vi "Dashboard Main.vi"() -> ()   [LabVIEW 2017]
uses:
  <vilib>/Utility/miscctls.llb/LVRowAndColumnTypeDef.ctl
  <vilib>/event_ctls.llb/eventvkey.ctl
  <vilib>/Rock Robotics/Network Tables/NT Read Numeric Array.vi
  <vilib>/Rock Robotics/WPI/Dashboard/WPI_DashboardLogging Global.vi
  <vilib>/Utility/config.llb/Read Key (Double).vi
  <vilib>/Utility/config.llb/Read Key (I32).vi
  <vilib>/Utility/config.llb/Write Key (Double).vi
  <vilib>/Utility/config.llb/Write Key (I32).vi
  <vilib>/Rock Robotics/Network Tables/NT Write Boolean.vi
  <vilib>/Utility/config.llb/NI_LVConfig.lvlib
panel:
  in  "Camera Settings Right":T1={"Frame Rate"=30, "Compression"=30, "Size"=1, "DB Camera Config"=FALSE} {"Frame Rate" scale=1.0..30.0; "Compression" scale=100.0..-1.0; "Size" items=["640x480", "320x240", "160x120"]}
  in  "Camera Name Right":string(combo)="No Camera Selection"
  out "Camera Info":cluster{"Mbps LED":bool, "Mbps":dbl, "fps":dbl} {"fps" format="%#.1g"; "Mbps" format="%#.1g"}
  in  "Camera Settings":T1={"Frame Rate"=30, "Compression"=30, "Size"=1, "DB Camera Config"=FALSE} {"Frame Rate" scale=1.0..30.0; "Compression" scale=100.0..-1.0; "Size" items=["640x480", "320x240", "160x120"]}
  in  "TCP":refnum<k5>
  in  "Rec Mode":enum32{"Stop", "Record", "Playback"}(radio)
  out "Robot IP":string
  out "Image Message":string="Timeout in Camera Communications"
  in  "Dashboard Tab":T2(tab)
  in  "DriveMode":T3(ring)
  in  "Autonomous":enum16{"CrossTheLine", "DoNothing"}(ring)
  in  "Encoders":T4(radio)
  in  "RobotPosition":T5(ring)
  in  "Gyro":bool
  in  "Boolean 2":bool
  in  "Select Auto":string(combo)="Select Autonomous ..."
  out "NT Connection":bool
  out "MotorChart R":cluster{"Numeric":dbl, "Numeric":dbl}(graph)
  out "MotorChart L":cluster{"Numeric":dbl, "Numeric":dbl}(graph)
  out "MotorSliders R":cluster{"MotorSlide1":dbl, "MotorSlide2":dbl} {"MotorSlide2" scale=-1.0..1.0 scale format="%#_2e"; "MotorSlide1" scale=-1.0..1.0 scale format="%#_2e"}
  out "MotorSliders L":cluster{"MotorSlide1":dbl, "MotorSlide2":dbl} {"MotorSlide2" scale=-1.0..1.0 scale format="%#_2e"; "MotorSlide1" scale=-1.0..1.0 scale format="%#_2e"}
  out "Gyro":dbl(knob) scale=0.0..360.0
  out "JS1 Z":dbl(slide) scale=-1.0..1.0 scale format="%#_2e"
  out "JS1 Graph":cluster{"X":dbl, "Y":dbl}[](graph)
  out "JS1 Buttons":T6
  out "JS2 Z":dbl(slide) scale=-1.0..1.0 scale format="%#_2e"
  out "JS2 Graph":cluster{"X":dbl, "Y":dbl}[](graph)
  out "JS2 Buttons":T6
  out "Mode":T7(ring)=enum."Auto Disabled"
  in  "ConfigFile":enum16{"Competition", "Sister", "DrivePractice"}(ring)
  out "Camera Image Right":T8(plugin-control)
  in  "Load":bool
  in  "Save":bool
  in  "DAutoGyro":dbl
  in  "IAutoGyro":dbl
  in  "PAutoGyro":dbl
  in  "FAutoGyro":dbl
  in  "RampRateAuto":dbl
  in  "FAutoRight":dbl
  in  "DAuto":dbl
  in  "IAuto":dbl
  in  "PAuto":dbl
  in  "FAutoLeft":dbl
  in  "DTeleGyro":dbl
  in  "ITeleGyro":dbl
  in  "PTeleGyro":dbl
  in  "RampRateTele":dbl
  in  "XYRatio":dbl
  in  "NormalPercent":dbl
  in  "TurboPercent":dbl
  in  "DriveMaxRPM":dbl
  in  "DTele":dbl
  in  "ITele":dbl
  in  "PTele":dbl
  in  "FTeleRight":dbl
  in  "FTeleLeft":dbl
  in  "FTeleGyro":dbl
  in  "Logging":bool
  in  "Test Slider":dbl(slide) scale=0.0..100.0 scale format="%#_3g"
  in  "On/Off":bool caption="Solenoid"
  in  "Test Name":u16(ring) items=["Select the test to run..."]
  in  "Test Tree":string(tree)
  in  "Motor":cluster{"Value":dbl, "Enable":bool} {"Value" scale=-1.0..1.0 scale format="%#_3g"}
  out "Progress":T9 {"Test Progress" scale=0.0..100.0}
  in  "Rev/Fwd":cluster{"Forward":bool, "Reverse":bool}
  in  "Test Ring":u16(ring) items=["Monochrome", "Color"]
  out "Cmd Status":string
  in  "Execute Command":bool
  in  "Command Params":string[][](table)
  in  "Command Selection":i32(listbox)
  in  "CheckList":i32(listbox)
  out "Tree":string(tree)
  out "Camera Image":T8(plugin-control)
  out "Background":bool
  in  "Camera Name":string(combo)="No Camera Selection"
  # "HW"
  # "HW"
  # "Joysticks"
  # "Front"
  # "Drive Motors"
  # "Right"
  # "Left"
  # "Back"
  # "This tab is a great place for autonomous settings and robot-specific values.\nPlace controls and indicators inside this tab and match name to\nDashboard Variables on robot. You can also delete this comment."
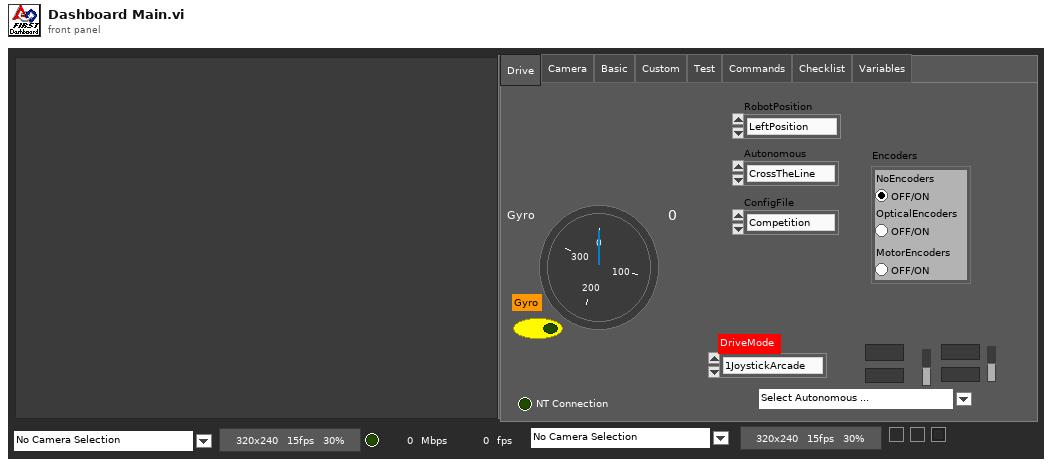
[diagram p1: front panel]
types:
  T1 = cluster{"Frame Rate":i32, "Compression":i32, "Size":u16, "DB Camera Config":bool}
  T2 = enum32{"Drive", "Camera", "Basic", "Custom", "Test", "Commands", "Checklist", "Variables"}
  T3 = enum16{"1JoystickArcade", "2JoystickArcade", "Tank"}
  T4 = enum32{"NoEncoders", "OpticalEncoders", "MotorEncoders"}
  T5 = enum16{"LeftPosition", "MiddlePosition", "RightPosition"}
  T6 = cluster{bool, bool, bool, bool, bool, bool, bool, bool, bool, bool, bool, bool}
  T7 = enum8{"Tele-Op Disabled", "Tele-Op Enabled", "Auto Disabled", "Auto Enabled", "Test Disabled", "Test Enabled", "Disconnected", "No Code", "E-Stop"}
  T8 = typedef "IMAQ Image.ctl" = refnum<image>
  T9 = cluster{"Test Progress":u8, "Test Progress Text":string}
  T10 = cluster{"Save Path":path, "Interval (s)":dbl, "Keep":i32}
  T11 = typedef "Image Type" = u32
  T12 = cluster{"IDs":cluster{"RPC field ID":u16, "Unique ID":u16}, "String":string}
  T13 = cluster{"Error Strings":string, "Disable Counts":cluster{u16, u16}, "Rail Faults":cluster{u16, u16, u16}, "Robot IP":string, "DB Mode":u8, "Event Info":cluster{"Name":string, "Type":u8, "Number":u16, "Replay":u8}}
  T14 = cluster{"Storage":cluster{"Disk Free":u64, "RAM Block":u32, "RAM free":u32}, "CPU Utilization":cluster{"CPU % ISR":sgl, "CPU % Time Crit":sgl, "CPU % Timed Str":sgl, "CPU % High":sgl, "CPU % Above":sgl, "CPU % Normal":sgl, "CPU % Low":sgl}, "CAN":cluster{"% Bus Utilization":sgl, "Bus Off Cnt":u32, "TX_FIFO Full Cnt":u32, "Receive Error Cnt":u8, "Transmit Error Cnt":u8}, "HID":cluster{"HID Outputs":u32, "Rumble Low":u16, "Rumble High":u16}[]}
  T15 = cluster{"Status bits":cluster{"Test Mode":bool, "Autonomous":bool, "Enabled":bool, "Code Start":bool, "Brownout":bool, "Reserved 2":bool, "Reserved 3":bool, "E-Stop":bool}, "Code Trace":cluster{"Disabled":bool, "TeleOp":bool, "Auto":bool, "Test":bool}, "Controller Type":enum16{"unknown", "cRIO", "roboRio"}, "Code?":enum16{"unknown", "noCode", "code"}, "Battery V":dbl}
  T16 = cluster{"Control Bits":cluster{"TestMode":bool, "Autonomous":bool, "Enabled":bool, "FMS Present":bool, bool, bool, bool, "E-Stop":bool}, "Team Station ":u8, "Countdown":sgl, "Joystick Values":cluster{"Axes":dbl[], "Buttons":bool[], "POVs":i16[]}[]}
  T17 = cluster{"Axes":dbl[], "Buttons":bool[], "POVs":i16[]}[]
  T18 = cluster{"Axes":dbl[], "Buttons":bool[], "POVs":i16[]}
  T19 = cluster{"Buttons[0]":bool, "Buttons[1]":bool, "Buttons[2]":bool, "Buttons[3]":bool, "Buttons[4]":bool, "Buttons[5]":bool, "Buttons[6]":bool, "Buttons[7]":bool, "Buttons[8]":bool, "Buttons[9]":bool, "Buttons[10]":bool, "Buttons[11]":bool}
  T20 = cluster{"Camera Name":string, string, "Saved DB Images Info":cluster{"Save Path":path, "Interval (s)":dbl, "Keep":i32}}
  T21 = cluster{"Camera Name Right":string, string, "Saved DB Images Info":cluster{"Save Path":path, "Interval (s)":dbl, "Keep":i32}}
  T22 = cluster{"Operation":enum16{"Update", "Clear"}, "Color Box":u32}[]
  T23 = typedef "eventvkey.ctl" = enum16{"ASCII", "Enter", "Return", "Shift", "Ctrl", "Alt", "Cmd", "Opt", "Caps", "NumLock", "Clear", "Break", "Up", "Down", "Left", "Right", "Insert", "Delete", "Home", "End", "PageUp", "PageDown", "Escape", "Help", "Pause", "ScrollLock", "F1", "F2", "F3", "F4", "F5", "F6", "F7", "F8", "F9", "F10", "F11", "F12", "F13", "F14", "F15", "F16", "F17", "F18", "F19", "F20", "F21", "F22", "F23", "F24", "Play", "VolumeUp", "VolumeDown", "Mute", "Two Byte Char"}
  T24 = cluster{"Image Size":bool, "Image Type":bool, "Pixel Value":bool, "ROI Information":bool, "Zoom Factor":bool}
  T25 = cluster{"Operation":enum16{"Update", "Clear"}, "Color Box":u32}
  T26 = typedef "LVRowAndColumnTypeDef.ctl" = cluster{"Row":i32, "Column":i32}
  T27 = cluster{"Shift":bool, "Ctrl":bool, "Alt":bool, "Cmd":bool, "Opt":bool}
  T28 = typedef "NI_LVConfig.lvlib/Config Data RefNum.ctl" = refnum<k1>
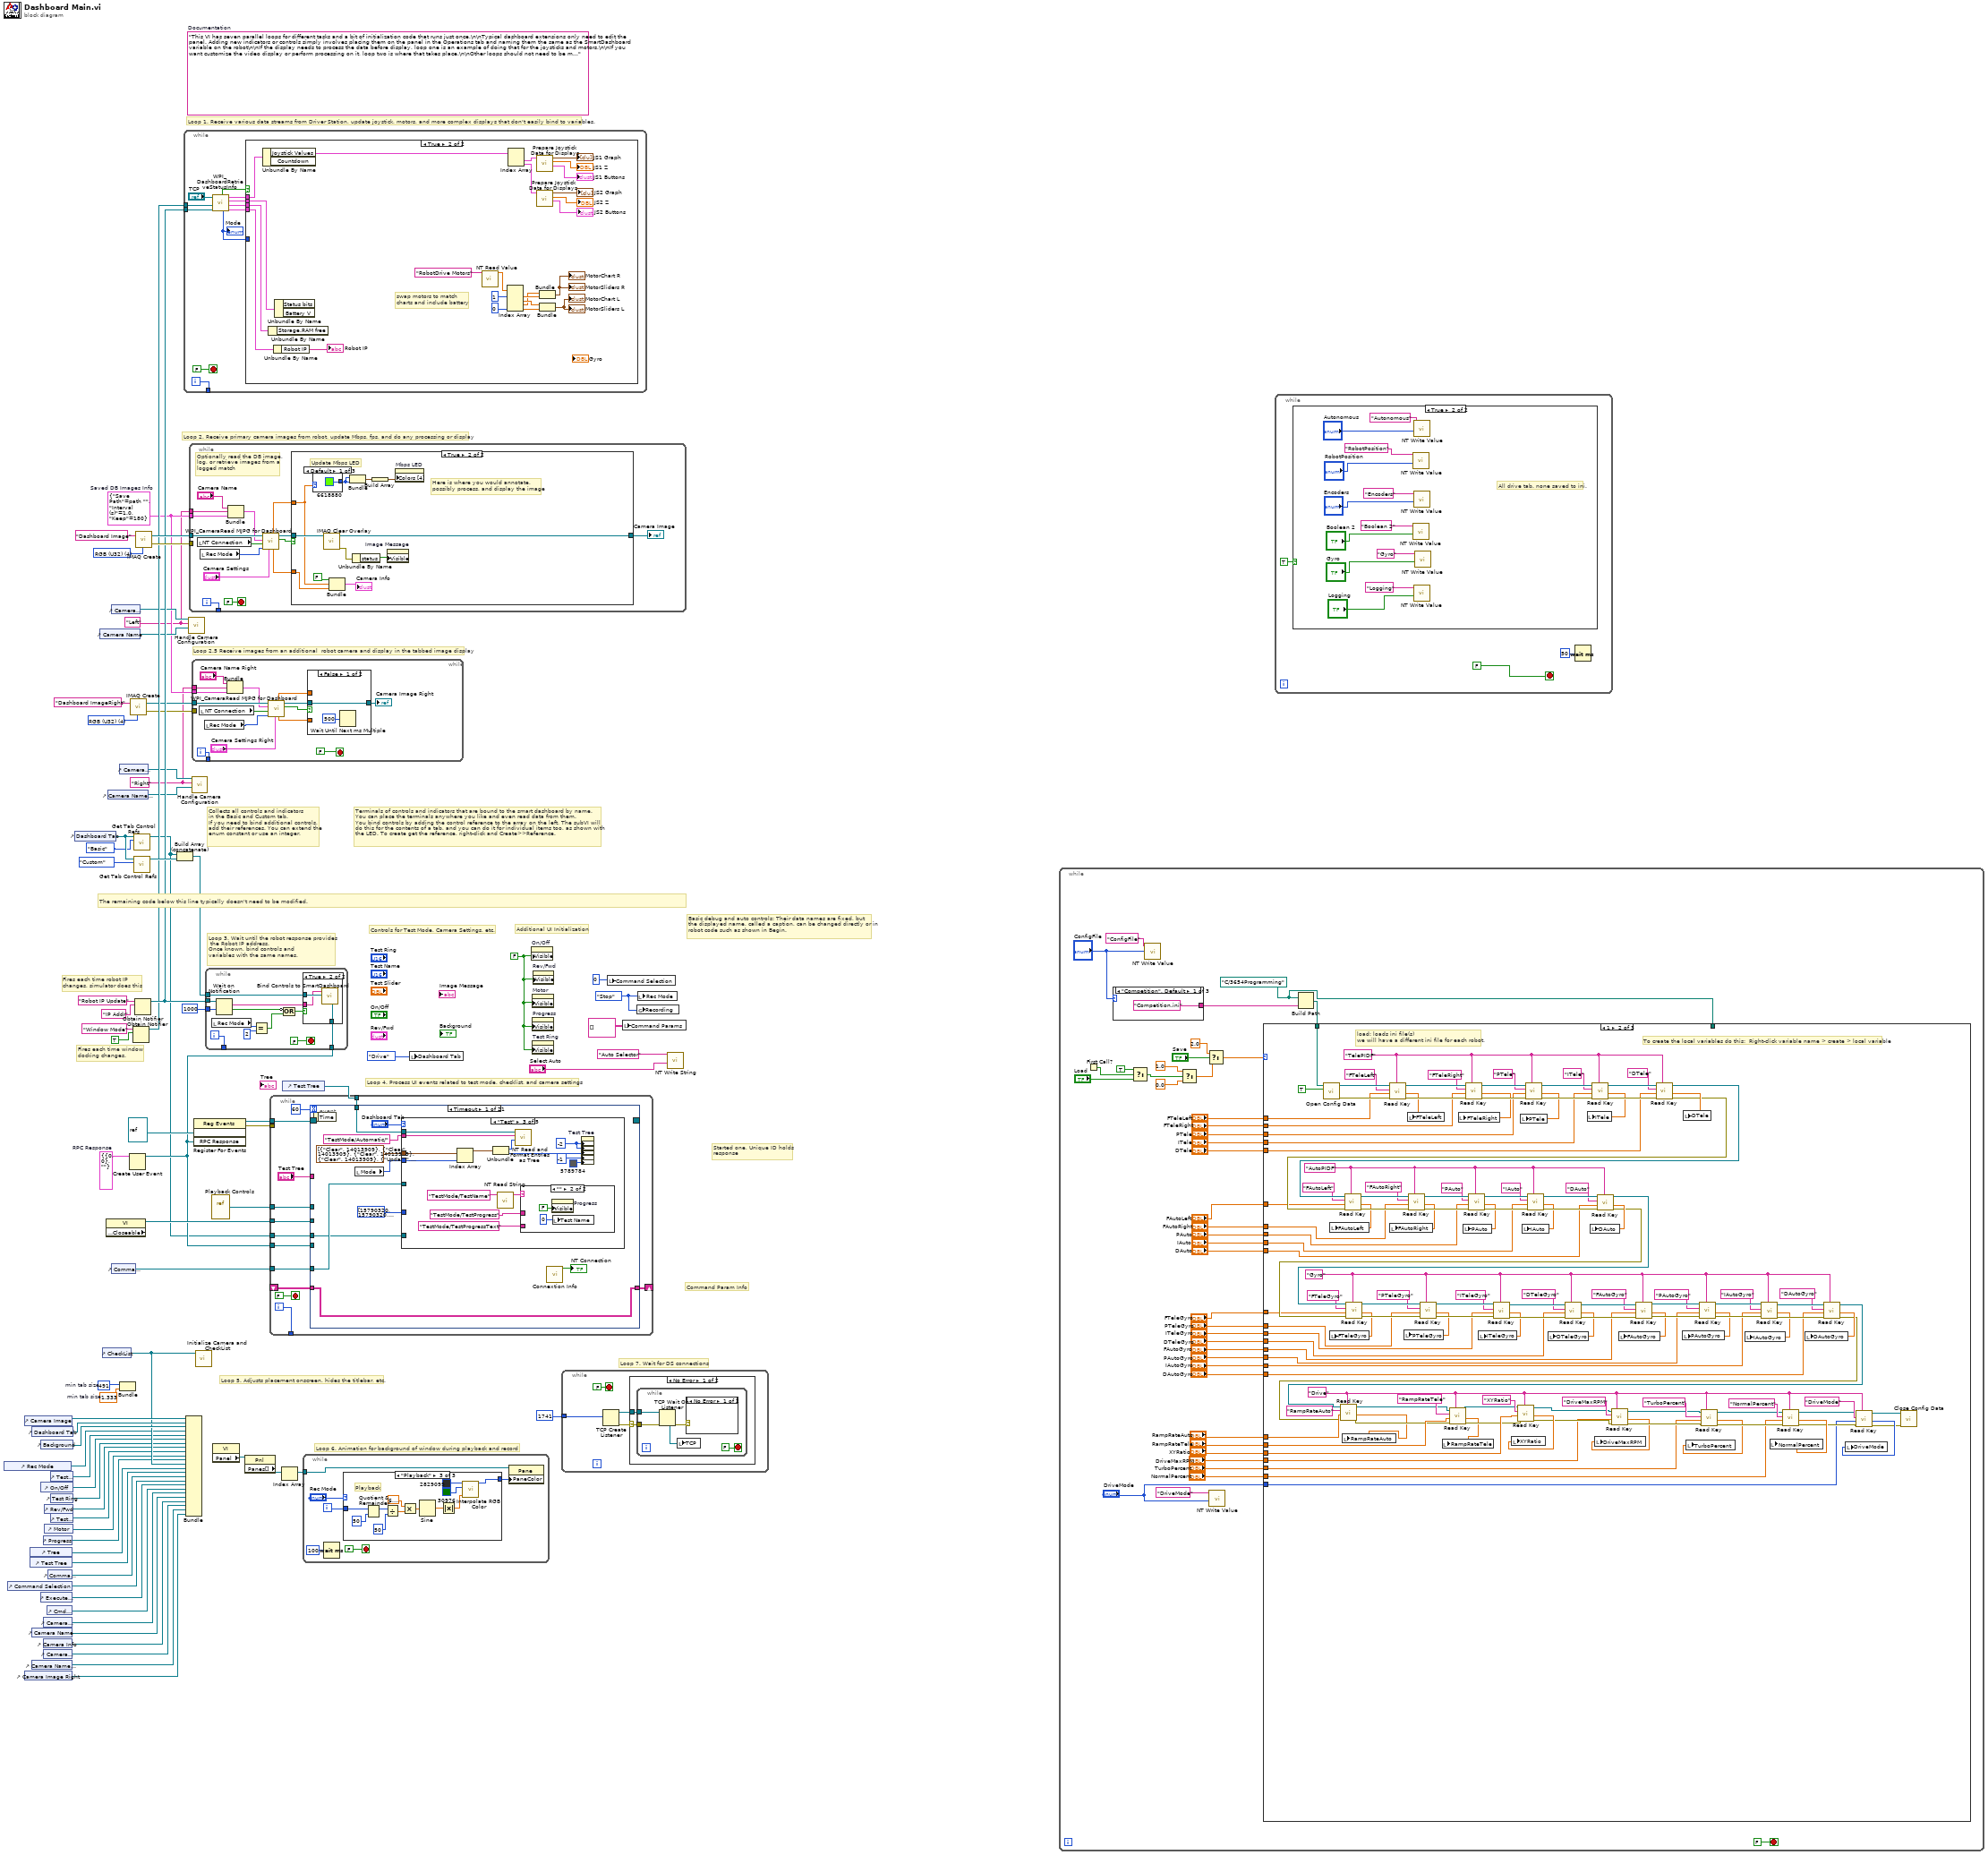
[diagram p0: block diagram]
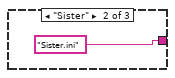
[diagram p3: hidden frame]
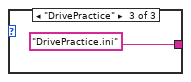
[diagram p4: hidden frame]
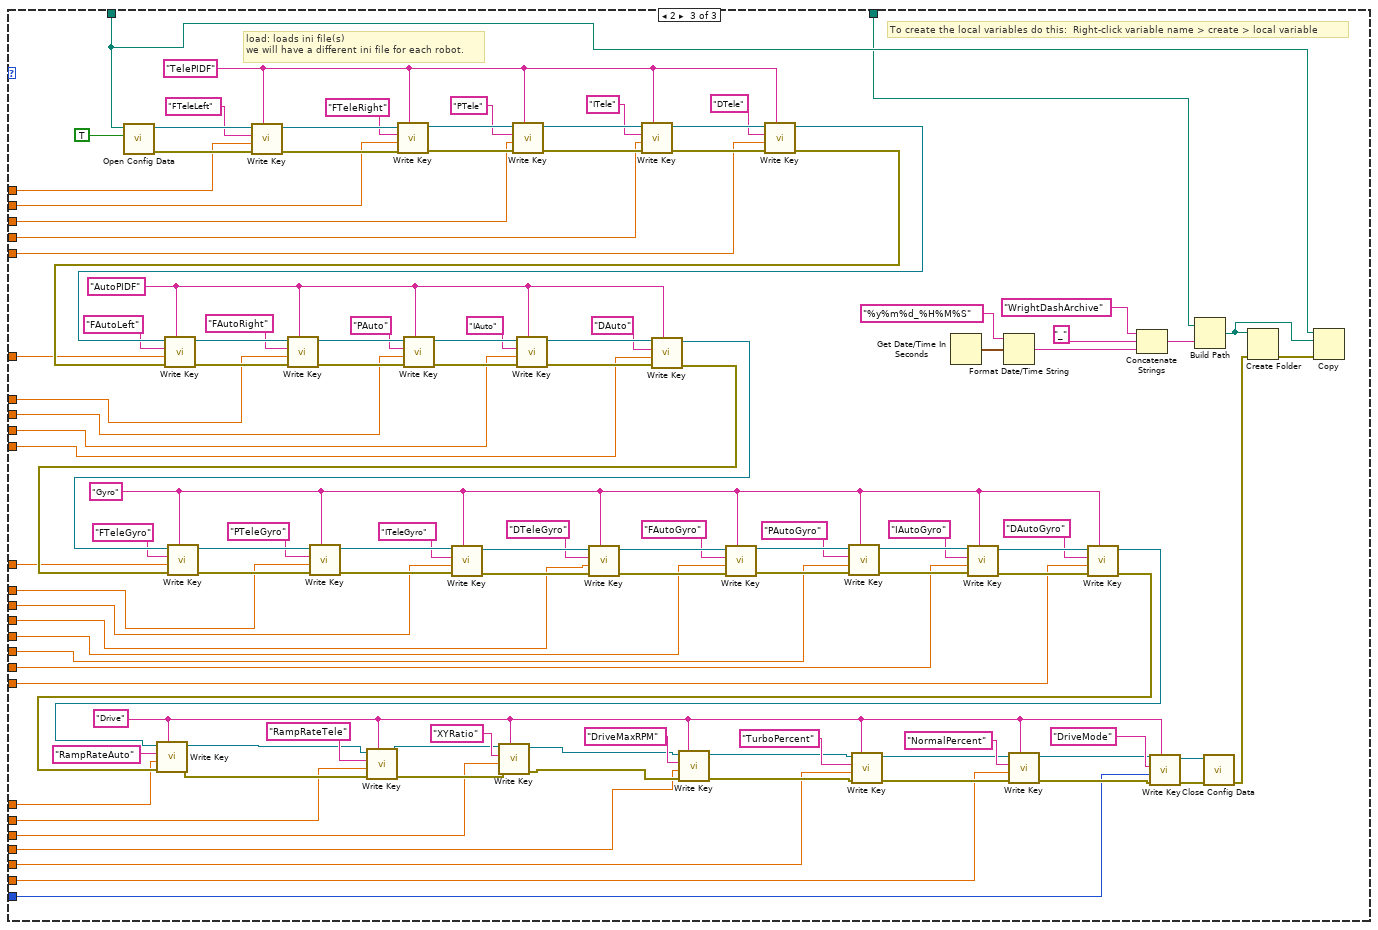
[diagram p6: hidden frame]
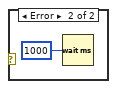
[diagram p8: hidden frame]
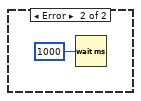
[diagram p9: hidden frame]
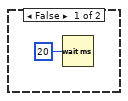
[diagram p10: hidden frame]
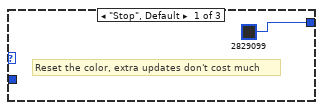
[diagram p11: hidden frame]
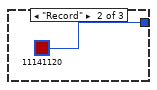
[diagram p12: hidden frame]
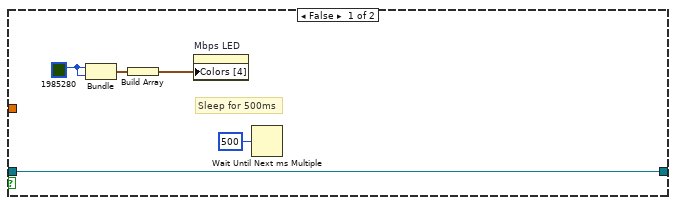
[diagram p14: hidden frame]
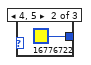
[diagram p15: hidden frame]
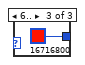
[diagram p16: hidden frame]
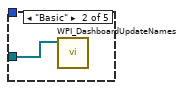
[diagram p18: hidden frame]
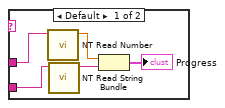
[diagram p19: hidden frame]
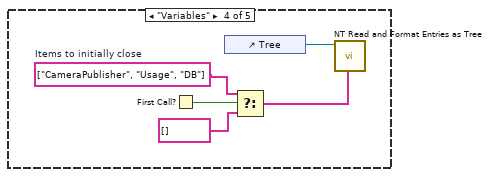
[diagram p20: hidden frame]
diagram:
  w3 = T10 {"Save Path"=path "", "Interval (s)"=1.0, "Keep"=180}  # Saved DB Images Info
  w2 = "Right"
  w1 = "Left"
  w13 = T11 4 items=["Grayscale (U8)", "Grayscale (I16)", "Grayscale (SGL)", "Complex (CSG)", "RGB (U32)", "HSL (U32)", "RGB (U64)"] ("Image Type")
  w29 = T12 {"IDs"={"RPC field ID"=0, "Unique ID"=0}, "String"=""}  # RPC Response
  w50 = 491  # min tab size
  w49 = 1.333  # min tab size
  w57 = enum32{"Stop", "Record", "Playback"}."Stop" ("Rec Mode")
  w36 = FALSE ("Visible")
  (unwired) "This VI has seven parallel loops for different tasks and a bit of initialization code that runs just once.\n\nTypical dashboard extensions only need to edit the panel. Adding new indicators or controls simply involves placing them on the panel in the Operations tab and naming them the same as the SmartDashboard variable on the robot\n\nIf the display needs to process the data before display, loop one is an example of doing that for the joysticks and motors.\n\nIf you want customize the video display or perform processing on it, loop two is where that takes place.\n\nOther loops should not need to be modified. They are pretty standard, and document the task they perform."  # Documentation
  w74 = T11 4 items=["Grayscale (U8)", "Grayscale (I16)", "Grayscale (SGL)", "Complex (CSG)", "RGB (U32)", "HSL (U32)", "RGB (U64)"] ("Image Type")
  # "Loop 2.5 Receive images from an additional  robot camera and display in the tabbed image display"
  # "Command Param Info"
  # "Started one, Unique ID holds\nresponse"
  # "Loop 7. Wait for DS connections"
  # "Basic debug and auto controls: Their data names are fixed, but\nthe displayed name, called a caption, can be changed directly or in\nrobot code such as shown in Begin."
  # "Controls for Test Mode, Camera Settings, etc."
  # "Additional UI Initialization"
  # "Loop 6. Animation for background of window during playback and record"
  # "Fires each time robot IP\nchanges, simulator does this"
  # "Fires each time window\ndocking changes."
  # "Collects all controls and indicators\nin the Basic and Custom tab.\nIf you need to bind additional controls,\nadd their references. You can extend the\nenum constant or use an integer."
  # "The remaining code below this line typically doesn't need to be modified."
  # "Loop 4. Process UI events related to test mode, checklist, and camera settings"
  # "Terminals of controls and indicators that are bound to the smart dashboard by name.\nYou can place the terminals anywhere you like and even read data from them.\nYou bind controls by adding the control reference to the array on the left. The subVI will\ndo this for the contents of a tab, and you can do it for individual items too, as shown with\nthe LED. To create get the reference, right-click and Create>>Reference."
  # "Loop 3. Wait until the robot response provides\n the Robot IP address.\nOnce known, bind controls and\nvariables with the same names."
  # "Loop 5. Adjusts placement onscreen, hides the titlebar, etc."
  # "Loop 1. Receive various data streams from Driver Station, update joystick, motors, and more complex displays that don't easily bind to variables."
  # "Loop 2. Receive primary camera images from robot, update Mbps, fps, and do any processing or display"
  n1 = control-ref of="Rec Mode"() -> (w42:refnum<vi>)
  n2 = control-ref of="Command Selection"() -> (w28:refnum<vi>)
  n3 = control-ref of="Camera Image Right"() -> (w6:refnum<vi>)
  n4 = control-ref of="Camera Image"() -> (w52:refnum<vi>)
  n5 = control-ref of="Tree"() -> (w46:refnum<vi>)
  n6 = control-ref of="Test Tree"() -> (w45:refnum<vi>)
  n7 = control-ref of="Dashboard Tab"() -> (w51:refnum<vi>)
  n8 = control-ref of="Camera Name"() -> (w19:refnum<vi>)
  n9 = control-ref of="Camera Name Right"() -> (w7:refnum<vi>)
  n10 = control-ref of="Execute Command"() -> (w30:refnum<vi>)
  n11 = control-ref of="Background"() -> (w48:refnum<vi>)
  n12 = control-ref of="On/Off"() -> (w40:refnum<vi>)
  n13 = control-ref of="Progress"() -> (w37:refnum<vi>)
  n14 = control-ref of="Camera Settings"() -> (w20:refnum<vi>)
  n15 = control-ref of="Camera Info"() -> (w18:refnum<vi>)
  n16 = control-ref of="Camera Settings Right"() -> (w8:refnum<vi>)
  n17 = control-ref of="Rev/Fwd"() -> (w38:refnum<vi>)
  n18 = control-ref of="Motor"() -> (w43:refnum<vi>)
  n19 = control-ref of="Cmd Status"() -> (w24:refnum<vi>)
  n20 = control-ref of="Command Params"() -> (w31:refnum<vi>)
  n21 = control-ref of="Test Slider"() -> (w41:refnum<vi>)
  n22 = control-ref of="Test Ring"() -> (w39:refnum<vi>)
  n23 = control-ref of="Test Name"() -> (w44:refnum<vi>)
  n24 = control-ref of="Dashboard Tab"() -> (w55:refnum<vi>)
  n25 = control-ref of="Camera Name"() -> (w21:refnum<vi>)
  n26 = control-ref of="CheckList"() -> (w47:refnum<vi>)
  n27 = property class="VI" props=["Front Panel.Closeable"]() -> (reference out=w56:refnum<vi>)  [unwired: 2 in, 2 out]
  n28 = control-ref of="Camera Name Right"() -> (w9:refnum<vi>)
  n29 = control-ref of="Camera Settings"() -> (w22:refnum<vi>)
  n30 = control-ref of="Command Params"() -> (w23:refnum<vi>)
  n31 = control-ref of="Camera Settings Right"() -> (w10:refnum<vi>)
  n32 = Bundle("min tab size"=w50, "min tab size"=w49) -> ()  [unwired: 1 in, 1 out]
  n33 = Create User Event(user event datatype=w29) -> (user event=w25:refnum<user-event>)  [unwired: 1 in, 1 out]
  n34 = call "IMAQ Create"("Image Name"="Dashboard ImageRight", "Image Type"=w13) -> ("New Image"=w12:T8, "error out"=w11:errorcluster)  [unwired: 2 in, 1 out]
  n35 = Obtain Notifier(name (unnamed)="Window Mode", notification data type=TRUE) -> (notifier out=w34:refnum<notifier>)  [unwired: 2 in, 2 out]
  n36 = call <vilib>:"Get Tab Control Refs.vi"("Page Index"=T2."Basic" ("Dashboard Tab"), "TabControl in"=w55) -> ("ControlsOnPage"=w17:refnum<vi>[])  [unwired: 9 in]
  n37 = call <vilib>:"Get Tab Control Refs.vi"("Page Index"=T2."Custom" ("Dashboard Tab"), "TabControl in"=w55) -> ("ControlsOnPage"=w54:refnum<vi>[])  [unwired: 9 in]
  n38 = Obtain Notifier(name (unnamed)="Robot IP Update", notification data type="IP Addr" ("name (unnamed)")) -> (notifier out=w35:refnum<notifier>)  [unwired: 2 in, 2 out]
  n39 = call "IMAQ Create"("Image Name"="Dashboard Image", "Image Type"=w74) -> ("New Image"=w72:T8, "error out"=w71:errorcluster)  [unwired: 2 in, 1 out]
  n40 = Build Array (concatenate)(w17, w54) -> (w53:refnum<vi>[])
  n41 = while {
    tunnel: [w84] -> _
    tunnel: w35 -> [w78]
    tunnel: w34 -> [w75]
    i -> [w84]
    stop <- FALSE stop-if-true
    n42 = call <vilib>:"WPI_DashboardRetrieveStatusInfo.vi"("Binding Refnum"=w78, "Window Mode Notifier"=w75, "TCP Cnx"="TCP") -> ("Power and Errors"=w79:T13, "Robot Metrics"=w82:T14, "Status Info"=w83:T15, "Control Info"=w80:T16, "Robot Mode"=w77:T7, "Process?"=w81:bool)  [unwired: 3 in]
    "Mode" <- w77
    n43 = case shown="True" w81 {
      tunnel: w83 -> [_ w110]
      tunnel: w82 -> [_ w109]
      tunnel: w80 -> [_ w108]
      tunnel: w79 -> [_ w107]
      tunnel: w77 -> [_ _]
      frame False {
        n44 = Wait (ms)(milliseconds to wait=u32 20) -> ()  [unwired: 1 out]
      }
      frame True {
        # "swap motors to match\ncharts and include battery"
        n45 = Unbundle By Name(w108) -> ("Joystick Values"=w98:T17)  [unwired: 1 out]
        n46 = Unbundle By Name(w109) -> ()  [unwired: 1 out]
        n47 = Unbundle By Name(w107) -> ("Robot IP"=→"Robot IP":string)
        n48 = Unbundle By Name(w110) -> ()  [unwired: 2 out]
        n49 = call-poly <vilib>:"NT Read Value.vi"("Name"="RobotDrive Motors") -> ("Numeric Array"=w88:dbl[])  [unwired: 9 in, 1 out]
        n50 = Index Array(array=w88, index #1=1, index #4=0) -> (element #1=w102:dbl, element #2=w103:dbl, element #3=w101:dbl, element #4=w106:dbl)  [unwired: 2 in]
        n51 = Index Array(array=w98) -> (element #1=w97:T18, element #2=w93:T18)  [unwired: 2 in]
        n52 = call "Prepare Joystick Data for Displays.vi"("Joystick Values"=w93) -> ("Buttons"=→"JS2 Buttons":T19, "Z Axis"=→"JS2 Z":dbl, "Cartesian Data"=→"JS2 Graph":cluster{"X axis":dbl, "X axis":dbl}[])  [unwired: 8 in]
        n53 = call "Prepare Joystick Data for Displays.vi"("Joystick Values"=w97) -> ("Buttons"=→"JS1 Buttons":T19, "Z Axis"=→"JS1 Z":dbl, "Cartesian Data"=→"JS1 Graph":cluster{"X axis":dbl, "X axis":dbl}[])  [unwired: 8 in]
        n54 = Bundle("Numeric"=w101, "Numeric"=w102) -> (→"MotorChart R" →"MotorSliders R":cluster{"Numeric":dbl, "Numeric":dbl})  [unwired: 1 in]
        n55 = Bundle("Numeric"=w103, "Numeric"=w106) -> (→"MotorChart L" →"MotorSliders L":cluster{"Numeric":dbl, "Numeric":dbl})  [unwired: 1 in]
      }
    }
  }
  n56 = Bundle("Camera Image"=w52, "Dashboard Tab"=w51, "Background"=w48, "Rec Mode"=w42, "Test Slider"=w41, "On/Off"=w40, "Test Ring"=w39, "Rev/Fwd"=w38, "Test Name"=w44, "Motor"=w43, "Progress"=w37, "CheckList"=w47, "Tree"=w46, "Test Tree"=w45, "Command Params"=w31, "Command Selection"=w28, "Execute Command"=w30, "Cmd Status"=w24, "Camera Settings"=w20, "Camera Name"=w19, "Camera Info"=w18, "Camera Settings Right"=w8, "Camera Name Right"=w7, "Camera Image Right"=w6) -> ()  [unwired: 1 in, 1 out]
  n57 = call "Handle Camera Configuration.vi"("CameraNameRef"=w21, "Display Name"=w1, "ClusterRef"=w22) -> ()  [unwired: 9 in]
  n58 = while {
    tunnel: w72 -> [w123]
    tunnel: w71 -> [_]
    tunnel: [w124] -> _
    tunnel: w3 -> [w114]
    tunnel: w1 -> [w111]
    i -> [w124]
    stop <- FALSE stop-if-true
    # "Optionally read the DB image,\nlog, or retrieve images from a\nlogged match"
    n59 = local read "NT Connection"() -> (w115:bool)
    n60 = local read "Rec Mode"() -> (w119:enum32{"Stop", "Record", "Playback"})
    n61 = Bundle("Camera Name"="Camera Name", w111, "Saved DB Images Info"=w114) -> (w113:T20)  [unwired: 1 in]
    n62 = call <vilib>:"WPI_CameraRead MJPG for Dashboard.vi"("Camera Settings"="Camera Settings", "Rec Mode"=w119, "NT Connection"=w115, "Capture Info"=w113, "Refnum in"=w123) -> ("Active"=w121:bool, "Refnum out"=w122:T8, "FPS"=w120:dbl, "Bandwidth (Mbps)"=w118:dbl)  [unwired: 3 in]
    n63 = case shown="True" w121 {
      tunnel: w122 -> [w126 w137]
      tunnel: w118 -> [_ w134]
      tunnel: w120 -> [_ w135]
      tunnel: [w126 w131] -> w116
      frame False {
        w128 = u32 1985280 ("Color Box")
        # "Sleep for 500ms"
        n64 = Bundle("Color Box"=w128, "Color Box"=w128) -> (w129:cluster{"Color Box":u32, "Color Box":u32})  [unwired: 1 out]
        n65 = Build Array(w129) -> (w127:cluster{"Color Box":u32, "Color Box":u32}[])
        n66 = property on="Mbps LED" class="Bool (strict)"("Colors [4]"=w127) -> ()  [unwired: 2 in, 2 out]
        n67 = Wait Until Next ms Multiple(millisecond multiple=u32 500) -> ()  [unwired: 1 out]
      }
      frame True {
        # "Here is where you would annotate,\npossibly process, and display the image"
        # "Update Mbps LED"
        n68 = case shown="Default" w134 {
          tunnel: [u32 6618880 ("Color Box") u32 16776722 ("Color Box") u32 16716800 ("Color Box")] -> w138
          frame Default {
          }
          frame 4, 5 {
          }
          frame 6.. {
          }
        }
        n69 = call "IMAQ Clear Overlay"("Image"=w137) -> ("error out"=w140:errorcluster, "Image Out"=w131:T8)  [unwired: 2 in, 7 out]
        n70 = Bundle(FALSE, "Bandwidth (Mbps)"=w134, "FPS"=w135) -> (→"Camera Info":cluster{bool, "Bandwidth (Mbps)":dbl, "FPS":dbl})  [unwired: 1 in]
        n71 = Bundle("Color Box"=w138, "Color Box"=w138) -> (w139:cluster{"Color Box":u32, "Color Box":u32})  [unwired: 1 out]
        n72 = Unbundle By Name(w140) -> ("status"=w141:bool)
        n73 = Build Array(w139) -> (w136:cluster{"Color Box":u32, "Color Box":u32}[])
        n74 = property on="Image Message" class="Str"("Visible"=w141) -> ()  [unwired: 2 in, 2 out]
        n75 = property on="Mbps LED" class="Bool (strict)"("Colors [4]"=w136) -> ()  [unwired: 2 in, 2 out]
      }
    }
    "Camera Image" <- w116
  }
  n76 = call "Handle Camera Configuration.vi"("CameraNameRef"=w9, "Display Name"=w2, "ClusterRef"=w10) -> ()  [unwired: 9 in]
  n77 = while {
    tunnel: w12 -> [w159]
    tunnel: w11 -> [_]
    tunnel: [w154] -> _
    tunnel: w3 -> [w148]
    tunnel: w2 -> [w145]
    i -> [w154]
    stop <- FALSE stop-if-true
    n78 = local read "NT Connection"() -> (w149:bool)
    n79 = local read "Rec Mode"() -> (w158:enum32{"Stop", "Record", "Playback"})
    n80 = Bundle("Camera Name Right"="Camera Name Right", w145, "Saved DB Images Info"=w148) -> (w147:T21)  [unwired: 1 in]
    n81 = call <vilib>:"WPI_CameraRead MJPG for Dashboard.vi"("Camera Settings"="Camera Settings Right", "Rec Mode"=w158, "NT Connection"=w149, "Capture Info"=w147, "Refnum in"=w159) -> ("Active"=w153:bool, "Refnum out"=w156:T8, "FPS"=w151:dbl, "Bandwidth (Mbps)"=w152:dbl)  [unwired: 3 in]
    n82 = case shown="False" w153 {
      tunnel: w156 -> [w160 w162]
      tunnel: w152 -> [_ _]
      tunnel: w151 -> [_ _]
      tunnel: [w160 w162] -> w150
      frame False {
        n83 = Wait Until Next ms Multiple(millisecond multiple=u32 500) -> ()  [unwired: 1 out]
      }
      frame True {
      }
    }
    "Camera Image Right" <- w150
  }
  n84 = register-events(refnum<vi> refnum, w25) -> (reference out=w61:refnum<event-registration>, error out=w60:errorcluster)  [unwired: 2 in]
  n85 = call "Initialize Camera and CheckList.vi"("ListBox in"=w47) -> ()  [unwired: 11 in]
  n86 = while {
    tunnel: w53 -> [w174]
    tunnel: w35 -> [w172]
    tunnel: [w170] -> _
    tunnel: u32 1000 ("milliseconds to wait") -> [w169]
    tunnel: w25 -> [w163]
    i -> [w170]
    stop <- FALSE stop-if-true
    n87 = local read "Rec Mode"() -> (w165:enum32{"Stop", "Record", "Playback"})
    n88 = Wait on Notification(notifier=w172, timeout in ms (-1)=w169) -> (notification=w171:string, timed out?=w167:bool)  [unwired: 2 in, 2 out]
    n89 = Equal?(x=w165, y=u16 2 ("Rec Mode")) -> (x = y?=w166:bool)
    n90 = Compound Arithmetic op=OR(invert w167, w166) -> (w168:bool)
    n91 = case shown="True" w168 {
      tunnel: w174 -> [_ w177]
      tunnel: w171 -> [_ w176]
      tunnel: w163 -> [_ w175]
      frame False {
      }
      frame True {
        n92 = call <vilib>:"Bind Controls to SmartDashboard.vi"("RPC ref"=w175, "Bound Control Refs"=w177, "Server IP Address"=w176) -> ()  [unwired: 9 in]
      }
    }
  }
  n93 = vi-ref "Playback Controls.vi"() -> (w62:refnum<vi>)
  n94 = property class="VI"() -> ("Panel"=w64:refnum<vi>)  [unwired: 2 in, 2 out]
  n95 = property class="Pnl"(reference=w64) -> ("Panes[]"=w65:refnum<vi>[])  [unwired: 1 in, 2 out]
  n96 = Index Array(array=w65) -> (element=w63:refnum<vi>)  [unwired: 1 in]
  n97 = control-ref of="Test Tree"() -> (w66:refnum<vi>)
  n98 = while {
    tunnel: [w187] -> _
    tunnel: w66 -> [w186]
    tunnel: w62 -> [w185]
    tunnel: w61 -> [w184]
    tunnel: w60 -> [_]
    tunnel: w56 -> [w183]
    tunnel: w25 -> [w182]
    tunnel: w23 -> [w181]
    shift-right: [w180] -> _
    shift-left: _ -> [w179]
    tunnel: w17 -> [w178]
    i -> [w187]
    stop <- FALSE stop-if-true
    n99 = event shown="[0] Timeout" {
      selector: w184 -> [_ _ _ _ _ _ _ _ _ _ _ _ _ _ _ _ _ _ _ _ _]
      dyn-events: [_ _ _ _ _ _ _ _ _ _ _ _ _ _ _ _ w447 _ _ _ _] -> _
      timeout: u32 60 ("milliseconds to wait") -> [_ _ _ _ _ _ _ _ _ _ _ _ _ _ _ _ _ _ _ _ _]
      tunnel: w186 -> [w199 _ _ _ _ _ _ _ _ _ _ _ _ _ _ _ _ _ _ _ _]
      tunnel: "Test Tree" -> [_ _ _ _ _ _ _ _ _ _ _ w414 w422 w424 w428 w436 _ _ _ _ _]
      tunnel: w185 -> [_ _ _ _ _ _ _ _ _ _ _ _ _ _ _ _ w449 _ w467 _ _]
      tunnel: w183 -> [_ _ _ _ _ _ _ _ _ _ _ _ _ _ _ _ w445 _ _ _ _]
      tunnel: w182 -> [_ _ _ _ _ _ _ _ _ _ _ _ _ _ _ _ w443 _ _ _ _]
      tunnel: w181 -> [w194 _ _ _ _ _ w365 _ _ _ _ _ _ _ _ _ _ _ _ _ _]
      tunnel: [w193 w242 w344 w349 w358 w362 w363 w372 w382 w389 w401 w413 w420 w423 w427 w435 w442 w462 w464 w468 w481] -> w180
      tunnel: w179 -> [w193 w242 w344 w349 w358 w362 w363 _ _ w389 w401 w413 w420 w423 w427 w435 w442 w462 w464 w468 w481]
      tunnel: w178 -> [w191 _ _ _ _ _ _ _ _ _ _ _ _ _ _ _ _ _ _ _ _]
      event Timeout {
        n100 = event-data() -> ()  [unwired: 1 in, 1 out]
        n101 = local read "Mode"() -> (w196:T7)
        n102 = case shown="\"Test\"" "Dashboard Tab" {
          tunnel: w199 -> [_ _ w215 _ _]
          tunnel: "TestMode/Automatic/" ("Name Pattern") -> [_ _ w214 _ _]
          tunnel: T22 [{"Operation"=enum."Clear", "Color Box"=14013909}, {"Operation"=enum."Clear", "Color Box"=14013909}, {"Operation"=enum."Clear", "Color Box"=14013909}, {"Operation"=enum."Clear", "Color Box"=14013909}, {"Operation"=enum."Update", "Color Box"=14013909}, {"Operation"=enum."Update", "Color Box"=16777215}, {"Operation"=enum."Clear", "Color Box"=14013909}, {"Operation"=enum."Clear", "Color Box"=14013909}, {"Operation"=enum."Clear", "Color Box"=14013909}] -> [_ _ w207 _ w235]
          tunnel: w196 -> [_ _ w206 _ w234]
          tunnel: u32[] [15790320, 15790320, 15790320, 15790320, 16777215, 16777215, 15790320, 15790320, 15790320] -> [_ _ _ _ w240]
          tunnel: w194 -> [_ _ _ _ w228]
          tunnel: w191 -> [_ w201 _ _ _]
          frame "Custom", Default {
          }
          frame "Basic" {
            n103 = call <vilib>:"WPI_DashboardUpdateNames.vi"("Controls on Tab"=w201) -> ()  [unwired: 11 in]
          }
          frame "Test" {
            w213 = -2 ("Active Item:Row Number")
            n104 = Index Array(array=w207, index=w206) -> (element=w208:T25)
            n105 = Unbundle(w208) -> ("Operation"=w209:enum16{"Update", "Clear"}, "Color Box"=w210:u32)
            n106 = call <vilib>:"NT Read String.vi"("Name"="TestMode/TestName") -> ("String"=w204:string)  [unwired: 9 in, 1 out]
            n107 = call <vilib>:"NT Read and Format Entries as Tree.vi"("Operation"=w209, "Name Pattern"=w214, "Tree Refnum"=w215) -> ()  [unwired: 7 in, 2 out]
            n108 = case shown="\"\"" w204 {
              tunnel: "TestMode/TestProgress" ("Name") -> [w217 _]
              tunnel: "TestMode/TestProgressText" ("Name") -> [w216 _]
              frame Default {
                n109 = call <vilib>:"NT Read Number.vi"("Name"=w217) -> ("Numeric"=w218:dbl)  [unwired: 9 in, 1 out]
                n110 = call <vilib>:"NT Read String.vi"("Name"=w216) -> ("String"=w219:string)  [unwired: 9 in, 1 out]
                n111 = Bundle("Numeric"=w218, "String"=w219) -> (→"Progress":cluster{"Numeric":dbl, "String":string})  [unwired: 1 in]
              }
              frame "" {
                n112 = property on="Progress" class="Clust (strict)"("Visible"=FALSE) -> ()  [unwired: 2 in, 2 out]
                n113 = local write "Test Name"(u16 0) -> ()
              }
            }
            n114 = property on="Test Tree" class="Tree (strict)"("Active Item Row Number"=w213, "ActiveColNum"=w213, "CellBG"=w210, "Active Item Row Number"=-1 ("Active Item:Row Number"), "CellBG"=u32 5789784 ("Color Box")) -> ()  [unwired: 2 in, 2 out]
          }
          frame "Variables" {
            w225 = string[] ["CameraPublisher", "Usage", "DB"]  # Items to initially close
            n115 = First Call?() -> (First Call?: T/F=w226:bool)
            n116 = control-ref of="Tree"() -> (w227:refnum<vi>)
            n117 = Select(t=w225, s=w226, f=string[] []) -> (s? t:f=w223:string[])
            n118 = call <vilib>:"NT Read and Format Entries as Tree.vi"("Tags to  Close"=w223, "Tree Refnum"=w227) -> ()  [unwired: 8 in, 2 out]
          }
          frame "Commands" {
            w236 = u32 5789784 ("Color Box")
            w237 = T26 {"Row"=-1, "Column"=-2} ("Active Cell:Active Cell")
            w239 = T26 {"Row"=-2, "Column"=-2} ("Active Cell:Active Cell")
            n119 = Index Array(array=w240, index=w234) -> (element=w238:u32)
            n120 = Index Array(array=w235, index=w234) -> (element=w233:T25)
            n121 = Unbundle(w233) -> ("Operation"=w232:enum16{"Update", "Clear"})  [unwired: 1 out]
            n122 = local read "Command Selection"() -> (w231:i32)
            n123 = property on="Command Selection" class="MCListbox (strict)"("ActiveCell"=w239, "CellBG"=w238, "ActiveCell"=w237, "CellBG"=w236) -> ()  [unwired: 2 in, 2 out]
            n124 = call <vilib>:"WPI_DashboardUpdate RPC Info.vi"("Operation"=w232) -> ("update"=w230:bool, "commands"=w229:string[][])  [unwired: 9 in]
            n125 = property on="Command Selection" class="MCListbox (strict)"("ItemNames"=w229) -> ()  [unwired: 2 in, 2 out]
            n126 = property on="Command Params" class="Tbl (strict)"("Active Cell"=w239, "Cell BG Color"=w238, "Active Cell"=w237, "Cell BG Color"=w236) -> ()  [unwired: 2 in, 2 out]
            n127 = call <vilib>:"WPI_DashboardUpdate Command Params.vi"("Update"=w230, "NewVal"=w231, "Commands"=w229, "Param Tbl"=w228) -> ()  [unwired: 7 in, 1 out]
          }
        }
        n128 = call <vilib>:"Connextion Info.vi"() -> ("Connected"=→"NT Connection":bool)  [unwired: 10 in, 1 out]
      }
      event "Test Tree": Value Change {
        # "Show appropriate\ncontrols"
        n129 = event-data() -> ("CtlRef"=w245:refnum<vi>, "NewVal"=w243:string)  [unwired: 1 in]
        n130 = call <vilib>:"WPI_UtilitiesGetTreeIOName.vi"("NewVal"=w243, "TreeControl in"=w245) -> ("I/O Name"=w246:string)  [unwired: 9 in]
        n131 = case shown="\"Camera\"" w246 {
          selector: w246 -> [_ w253 _ w275 w284 _]
          tunnel: w243 -> [_ _ w272 w274 _ w291]
          tunnel: cluster{string[]}[] [{["640x480", "320x240", "160x120"]}, {["Auto", "Fixed indoor", "Fixed outdoor 1", "Fixed outdoor 2", "Fixed fluorescent 1", "Fixed fluorescent 2", "Hold current"]}, {["Auto", "Flicker-free 50 Hz", "Flicker-free 60 Hz", "Hold current"]}, {["None", "Prioritize frame rate", "Prioritize image quality"]}, {["Monochrome", "Color"]}] -> [_ _ _ _ _ w290]
          frame Default {
            w248 = FALSE ("Visible")
            w247 = FALSE ("Visible")
            n132 = property on="Motor" class="Clust (strict)"("Visible"=w247) -> ()  [unwired: 2 in, 2 out]
            n133 = property on="Test Ring" class="Ring (strict)"("Visible"=w247) -> ()  [unwired: 2 in, 2 out]
            n134 = property on="Rev/Fwd" class="Clust (strict)"("Visible"=w248) -> ()  [unwired: 2 in, 2 out]
            n135 = property on="On/Off" class="Bool (strict)"("Visible"=w248) -> ()  [unwired: 2 in, 2 out]
            n136 = property on="Test Slider" class="Slide (strict)"("Visible"=w248) -> ()  [unwired: 2 in, 2 out]
          }
          frame "Analog Out", "Motor", "PWM" {
            w254 = FALSE ("Visible")
            n137 = case shown="\"Analog Out\"" w253 {
              tunnel: [1.0 ("Value") -1.0 ("Value") 0.0 ("Value")] -> w252
              tunnel: [255.0 ("Value") 1.0 ("Value") 5.0 ("Value")] -> w251
              tunnel: [128.0 ("Value") 0.0 ("Value") 0.0 ("Value")] -> w250
              tunnel: [64.0 ("Value") 0.5 ("Value") 1.0 ("Value")] -> w249
              frame "PWM" {
              }
              frame "Motor", Default {
              }
              frame "Analog Out" {
              }
            }
            n138 = property on="Motor" class="Clust (strict)"("Visible"=TRUE) -> ()  [unwired: 2 in, 2 out]
            n139 = property on="Value" class="Slide (strict)"("Value"=w250, "Scale.Minimum"=w252, "Scale.Maximum"=w251, "Scale.Increment"=w249) -> ()  [unwired: 2 in, 2 out]
            n140 = property on="On/Off" class="Bool (strict)"("Visible"=w254) -> ()  [unwired: 2 in, 2 out]
            n141 = property on="Test Slider" class="Slide (strict)"("Visible"=w254) -> ()  [unwired: 2 in, 2 out]
            n142 = property on="Test Ring" class="Ring (strict)"("Visible"=w254) -> ()  [unwired: 2 in, 2 out]
            n143 = property on="Rev/Fwd" class="Clust (strict)"("Visible"=w254) -> ()  [unwired: 2 in, 2 out]
          }
          frame "Servo" {
            w270 = FALSE ("Visible")
            n144 = call <vilib>:"NT Read Number.vi"("Name"=w272) -> ("Numeric"=w271:dbl)  [unwired: 9 in, 1 out]
            n145 = property on="Test Slider" class="Slide (strict)"("Visible"=TRUE, "Scale.Maximum"=170.0 ("Scale.Range:Maximum")) -> ()  [unwired: 2 in, 2 out]
            n146 = local write "Test Slider"(w271) -> ()
            n147 = property on="Motor" class="Clust (strict)"("Visible"=w270) -> ()  [unwired: 2 in, 2 out]
            n148 = property on="Rev/Fwd" class="Clust (strict)"("Visible"=w270) -> ()  [unwired: 2 in, 2 out]
            n149 = property on="On/Off" class="Bool (strict)"("Visible"=w270) -> ()  [unwired: 2 in, 2 out]
            n150 = property on="Test Ring" class="Ring (strict)"("Visible"=w270) -> ()  [unwired: 2 in, 2 out]
          }
          frame "Relay", "Solenoid" {
            w273 = FALSE ("Visible")
            n151 = property on="Motor" class="Clust (strict)"("Visible"=w273) -> ()  [unwired: 2 in, 2 out]
            n152 = property on="Test Slider" class="Slide (strict)"("Visible"=w273) -> ()  [unwired: 2 in, 2 out]
            n153 = Search and Replace String(input string=w274, search string="/Value  **", replace string="/Direction") -> (result string=w280:string)  [unwired: 5 in, 3 out]
            n154 = property on="Test Ring" class="Ring (strict)"("Visible"=w273) -> ()  [unwired: 2 in, 2 out]
            n155 = call <vilib>:"NT Read String.vi"("Name"=w280) -> ("String"=w278:string)  [unwired: 9 in, 1 out]
            n156 = Equal?(x="Both directions", y=w278) -> (x = y?=w276:bool)
            n157 = Not(x=w276) -> (.not. x?=w277:bool)
            n158 = property on="Rev/Fwd" class="Clust (strict)"("Visible"=w276) -> ()  [unwired: 2 in, 2 out]
            n159 = property on="On/Off" class="Bool (strict)"("Visible"=w277, "Caption.Text"=w275) -> ()  [unwired: 2 in, 2 out]
          }
          frame "Compressor", "Digital Out" {
            w283 = FALSE ("Visible")
            # "Get direction and finish"
            n160 = property on="Motor" class="Clust (strict)"("Visible"=w283) -> ()  [unwired: 2 in, 2 out]
            n161 = property on="Test Slider" class="Slide (strict)"("Visible"=w283) -> ()  [unwired: 2 in, 2 out]
            n162 = property on="Test Ring" class="Ring (strict)"("Visible"=w283) -> ()  [unwired: 2 in, 2 out]
            n163 = property on="On/Off" class="Bool (strict)"("Visible"=TRUE, "Caption.Text"=w284) -> ()  [unwired: 2 in, 2 out]
            n164 = property on="Rev/Fwd" class="Clust (strict)"("Visible"=FALSE) -> ()  [unwired: 2 in, 2 out]
          }
          frame "Camera" {
            n165 = call <vilib>:"Get Last Path Segment.vi"("String in"=w291) -> ("String out"=w292:string)  [unwired: 10 in]
            n166 = property on="On/Off" class="Bool (strict)"("Visible"=FALSE) -> ()  [unwired: 2 in, 2 out]
            n167 = property on="Motor" class="Clust (strict)"("Visible"=FALSE) -> ()  [unwired: 2 in, 2 out]
            n168 = property on="Rev/Fwd" class="Clust (strict)"("Visible"=FALSE) -> ()  [unwired: 2 in, 2 out]
            n169 = case shown="\"White Balance  **\"" w292 {
              tunnel: w291 -> [w298 w307 w316 w325 w334 _ w340]
              tunnel: w290 -> [w296 w304 w313 w322 w331 _ _]
              frame "Size  **" {
                n170 = Index Array(array=w296) -> (element=w295:cluster{string[]})  [unwired: 1 in]
                n171 = call <vilib>:"NT Read String.vi"("Name"=w298) -> ("String"=w297:string)  [unwired: 9 in, 1 out]
                n172 = Unbundle(w295) -> (w293:string[])
                n173 = Match First String(2:w293, 3:w297) -> (0:w294:i32)  [unwired: 1 out]
                n174 = property on="Test Ring" class="Ring (strict)"("Value"=w294, "Strings []"=w293) -> ()  [unwired: 2 in, 2 out]
                n175 = property on="Test Ring" class="Ring (strict)"("Visible"=TRUE) -> ()  [unwired: 2 in, 2 out]
                n176 = property on="Test Slider" class="Slide (strict)"("Visible"=FALSE) -> ()  [unwired: 2 in, 2 out]
              }
              frame "White Balance  **" {
                n177 = Index Array(array=w304, index=1) -> (element=w305:cluster{string[]})
                n178 = call <vilib>:"NT Read String.vi"("Name"=w307) -> ("String"=w306:string)  [unwired: 9 in, 1 out]
                n179 = Unbundle(w305) -> (w302:string[])
                n180 = Match First String(2:w302, 3:w306) -> (0:w301:i32)  [unwired: 1 out]
                n181 = property on="Test Ring" class="Ring (strict)"("Value"=w301, "Strings []"=w302) -> ()  [unwired: 2 in, 2 out]
                n182 = property on="Test Ring" class="Ring (strict)"("Visible"=TRUE) -> ()  [unwired: 2 in, 2 out]
                n183 = property on="Test Slider" class="Slide (strict)"("Visible"=FALSE) -> ()  [unwired: 2 in, 2 out]
              }
              frame "Exposure  **" {
                n184 = Index Array(array=w313, index=2) -> (element=w314:cluster{string[]})
                n185 = call <vilib>:"NT Read String.vi"("Name"=w316) -> ("String"=w315:string)  [unwired: 9 in, 1 out]
                n186 = Unbundle(w314) -> (w310:string[])
                n187 = Match First String(2:w310, 3:w315) -> (0:w311:i32)  [unwired: 1 out]
                n188 = property on="Test Ring" class="Ring (strict)"("Value"=w311, "Strings []"=w310) -> ()  [unwired: 2 in, 2 out]
                n189 = property on="Test Ring" class="Ring (strict)"("Visible"=TRUE) -> ()  [unwired: 2 in, 2 out]
                n190 = property on="Test Slider" class="Slide (strict)"("Visible"=FALSE) -> ()  [unwired: 2 in, 2 out]
              }
              frame "Exposure Priority  **" {
                n191 = Index Array(array=w322, index=3) -> (element=w323:cluster{string[]})
                n192 = call <vilib>:"NT Read String.vi"("Name"=w325) -> ("String"=w324:string)  [unwired: 9 in, 1 out]
                n193 = Unbundle(w323) -> (w319:string[])
                n194 = Match First String(2:w319, 3:w324) -> (0:w320:i32)  [unwired: 1 out]
                n195 = property on="Test Ring" class="Ring (strict)"("Value"=w320, "Strings []"=w319) -> ()  [unwired: 2 in, 2 out]
                n196 = property on="Test Ring" class="Ring (strict)"("Visible"=TRUE) -> ()  [unwired: 2 in, 2 out]
                n197 = property on="Test Slider" class="Slide (strict)"("Visible"=FALSE) -> ()  [unwired: 2 in, 2 out]
              }
              frame "Color Enable  **" {
                n198 = Index Array(array=w331, index=4) -> (element=w332:cluster{string[]})
                n199 = call <vilib>:"NT Read String.vi"("Name"=w334) -> ("String"=w333:string)  [unwired: 9 in, 1 out]
                n200 = Unbundle(w332) -> (w328:string[])
                n201 = Match First String(2:w328, 3:w333) -> (0:w329:i32)  [unwired: 1 out]
                n202 = property on="Test Ring" class="Ring (strict)"("Value"=w329, "Strings []"=w328) -> ()  [unwired: 2 in, 2 out]
                n203 = property on="Test Ring" class="Ring (strict)"("Visible"=TRUE) -> ()  [unwired: 2 in, 2 out]
                n204 = property on="Test Slider" class="Slide (strict)"("Visible"=FALSE) -> ()  [unwired: 2 in, 2 out]
              }
              frame Default {
                n205 = property on="Test Ring" class="Ring (strict)"("Visible"=FALSE) -> ()  [unwired: 2 in, 2 out]
                n206 = property on="Test Slider" class="Slide (strict)"("Visible"=FALSE) -> ()  [unwired: 2 in, 2 out]
              }
              frame "Brightness  **", "Color Level  **", "Compression  **", "FPS  **", "Sharpness  **" {
                n207 = call <vilib>:"NT Read Number.vi"("Name"=w340) -> ("Numeric"=w339:dbl)  [unwired: 9 in, 1 out]
                n208 = local write "Test Slider"(w339) -> ()
                n209 = property on="Test Slider" class="Slide (strict)"("Visible"=TRUE, "Scale.Maximum"=100.0 ("Scale.Range:Maximum")) -> ()  [unwired: 2 in, 2 out]
                n210 = property on="Test Ring" class="Ring (strict)"("Visible"=FALSE) -> ()  [unwired: 2 in, 2 out]
              }
            }
          }
        }
        n211 = property on="Progress" class="Clust (strict)"("Visible"=FALSE) -> ()  [unwired: 2 in, 2 out]
      }
      event "Test Name": Mouse Enter {
        # "Populate the ring with the list of tests"
        n212 = event-data() -> ()  [unwired: 1 in, 1 out]
        n213 = call <vilib>:"NT Read String Array.vi"("Name"="TestMode/TestList") -> ("String Array"=w348:string[])  [unwired: 9 in, 1 out]
        n214 = Build Array (concatenate)("Select the test to run...", w348) -> (w347:string[])
        n215 = property on="Test Name" class="Ring (strict)"("Strings []"=w347) -> ()  [unwired: 2 in, 2 out]
      }
      event "Test Name": Value Change {
        w350 = FALSE ("Visible")
        # "Tell the robot the test name to run"
        n216 = event-data() -> ("NewVal"=w354:u16)  [unwired: 1 in]
        n217 = property on="Test Name" class="Ring (strict)"() -> ("Strings []"=w355:string[])  [unwired: 2 in, 2 out]
        n218 = local write "Progress"(T9 {"Test Progress"=0, "Test Progress Text"=""} ("Progress")) -> ()
        n219 = Index Array(array=w355, index=w354) -> (element=w353:string)
        n220 = call <vilib>:"NT Write String.vi"("String"=w353, "Name"="TestMode/TestName") -> ()  [unwired: 9 in, 1 out]
        n221 = property on="Progress" class="Clust (strict)"("Visible"=TRUE) -> ()  [unwired: 2 in, 2 out]
        n222 = property on="Motor" class="Clust (strict)"("Visible"=w350) -> ()  [unwired: 2 in, 2 out]
        n223 = property on="Test Slider" class="Slide (strict)"("Visible"=w350) -> ()  [unwired: 2 in, 2 out]
        n224 = property on="On/Off" class="Bool (strict)"("Visible"=w350) -> ()  [unwired: 2 in, 2 out]
        n225 = property on="Rev/Fwd" class="Clust (strict)"("Visible"=w350) -> ()  [unwired: 2 in, 2 out]
        n226 = property on="Test Ring" class="Ring (strict)"("Visible"=w350) -> ()  [unwired: 2 in, 2 out]
      }
      event "Select Auto": Mouse Enter {
        # "Populate the combo box with the list of autonomous options"
        n227 = event-data() -> ()  [unwired: 1 in, 1 out]
        n228 = call <vilib>:"NT Read String Array.vi"("Name"="Auto List") -> ("String Array"=w357:string[])  [unwired: 9 in, 1 out]
        n229 = property on="Select Auto" class="CmbBox"("Strings[]"=w357) -> ()  [unwired: 2 in, 2 out]
      }
      event "Select Auto": Value Change {
        # "User modified the Auto Selection. Write to NT variable so robot knows."
        n230 = event-data() -> ("NewVal"=w360:string)  [unwired: 1 in]
        n231 = call <vilib>:"NT Write String.vi"("String"=w360, "Name"="Auto Selector") -> ()  [unwired: 9 in, 1 out]
      }
      event "Command Selection": Value Change {
        # "Get the params and show in table"
        n232 = event-data() -> ("NewVal"=w366:i32)  [unwired: 1 in]
        n233 = property on="Command Selection" class="MCListbox (strict)"() -> ("ItemNames"=w364:string[][])  [unwired: 2 in, 2 out]
        n234 = call <vilib>:"WPI_DashboardUpdate Command Params.vi"("NewVal"=w366, "Commands"=w364, "Param Tbl"=w365) -> ()  [unwired: 8 in, 1 out]
      }
      event "Execute Command": Value Change {
        # "Started one, Unique ID holds\nresponse"
        n235 = event-data() -> ()  [unwired: 1 in, 1 out]
        n236 = property on="Command Selection" class="MCListbox (strict)"() -> ("ItemNames"=w377:string[][])  [unwired: 2 in, 2 out]
        n237 = Index Array(array=w377, index (row)="Command Selection", index (col)=0) -> (element=w375:string)
        n238 = call <vilib>:"Invoke Commands.vi"("Command Params"="Command Params", "Function Name"=w375) -> ("Params"=w371:u8, "Started"=w370:bool)  [unwired: 7 in, 1 out]
        n239 = Array Subset(array="Command Params", length (row)=w371) -> (w372:string[][])  [unwired: 3 in]
        n240 = Select(t="Executing" ("Cmd Status"), s=w370, f="" ("Cmd Status")) -> (s? t:f=→"Cmd Status":string)
      }
      event "Command Selection": Double Click {
        n241 = event-data() -> ("Row"=w385:i32)  [unwired: 1 in]
        n242 = property on="Command Selection" class="MCListbox (strict)"() -> ("ItemNames"=w388:string[][])  [unwired: 2 in, 2 out]
        n243 = local read "Command Params"() -> (w384:string[][])
        n244 = Index Array(array=w388, index (row)=w385, index (col)=0) -> (element=w386:string)
        n245 = call <vilib>:"Invoke Commands.vi"("Command Params"=w384, "Function Name"=w386) -> ("Params"=w383:u8, "Started"=w378:bool)  [unwired: 7 in, 1 out]
        n246 = Array Subset(array=w384, length (row)=w383) -> (w382:string[][])  [unwired: 3 in]
        n247 = Select(t="Executing" ("Cmd Status"), s=w378, f="" ("Cmd Status")) -> (s? t:f=w379:string)
        n248 = local write "Cmd Status"(w379) -> ()
      }
      event "CheckList": Double Click {
        # "Shift clears all"
        # "Update symbols on the listbox"
        n249 = event-data() -> ("PlatMods.Shift"=w390:bool, "Row"=w392:i32)  [unwired: 1 in]
        n250 = case shown="True" w390 {
          tunnel: w392 -> [w396 _]
          tunnel: 1 -> [w395 _]
          frame False {
            n251 = property on="CheckList" class="LstBox (strict)"() -> ("Item Symbols"=w394:i32[])  [unwired: 2 in, 2 out]
            n252 = Replace Array Subset(array=w394, new element=w395, index=w396) -> (w393:i32[])
            n253 = property on="CheckList" class="LstBox (strict)"("Item Symbols"=w393) -> ()  [unwired: 2 in, 2 out]
          }
          frame True {
            w397 = 0 ("Top Row")
            n254 = property on="CheckList" class="LstBox (strict)"() -> ("Number of Rows"=w399:u32)  [unwired: 2 in, 2 out]
            n255 = Initialize Array(0, w399) -> (w398:i32[])
            n256 = property on="CheckList" class="LstBox (strict)"("Top Row"=w397, "Value"=w397, "Item Symbols"=w398) -> ()  [unwired: 2 in, 2 out]
          }
        }
      }
      event "CheckList": Key Down {
        # "Update symbols on the listbox\nLeft and right keys check and uncheck"
        n257 = event-data() -> ("VKey"=w403:T23)  [unwired: 1 in]
        n258 = case shown="\"Left\", \"Right\"" w403 {
          selector: w403 -> [w408 _]
          tunnel: eventvkey."Left" ("VKey") -> [w406 _]
          frame "Left", "Right" {
            n259 = Equal?(x=w406, y=w408) -> (x = y?=w407:bool)
            n260 = Select(t=0, s=w407, f=1) -> (s? t:f=w409:i32)
            n261 = property on="CheckList" class="LstBox (strict)"() -> ("Item Symbols"=w412:i32[])  [unwired: 2 in, 2 out]
            n262 = Replace Array Subset(array=w412, new element=w409, index="CheckList") -> (w411:i32[])
            n263 = property on="CheckList" class="LstBox (strict)"("Item Symbols"=w411) -> ()  [unwired: 2 in, 2 out]
          }
          frame Default {
          }
        }
      }
      event "Motor.Enable": Value Change {
        # "When the test mode otor enable helper is set, update that\ntree row item's value"
        n264 = event-data() -> ("NewVal"=w418:bool)  [unwired: 1 in]
        n265 = Unbundle("Motor") -> ("Value"=w417:dbl)  [unwired: 1 out]
        n266 = Select(t=w417, s=w418, f=0.0) -> (s? t:f=w415:dbl)
        n267 = call <vilib>:"NT Write Number.vi"("Numeric"=w415, "Name"=w414) -> ()  [unwired: 9 in, 1 out]
      }
      event "Test Slider": Value Change {
        # "When the test mode slider helper is set, update that\ntree row item's value"
        n268 = event-data() -> ("NewVal"=w421:dbl)  [unwired: 1 in]
        n269 = call <vilib>:"NT Write Number.vi"("Numeric"=w421, "Name"=w422) -> ()  [unwired: 9 in, 1 out]
      }
      event "On/Off": Value Change {
        # "When the test mode on/off helper value is set, update that\ntree row item's value"
        n270 = event-data() -> ("NewVal"=w426:bool)  [unwired: 1 in]
        n271 = Boolean To (0,1)(Boolean=w426) -> (0, 1=w425:i16)
        n272 = call <vilib>:"NT Write Number.vi"("Numeric"=w425, "Name"=w424) -> ()  [unwired: 9 in, 1 out]
      }
      event "Rev/Fwd": Value Change {
        # "When the test mode helper value for relays is set, update that\ntree row item's value"
        n273 = event-data() -> ("NewVal.Forward"=w434:bool, "NewVal.Reverse"=w433:bool)  [unwired: 1 in]
        n274 = Boolean To (0,1)(Boolean=w434) -> (0, 1=w430:i16)
        n275 = Boolean To (0,1)(Boolean=w433) -> (0, 1=w432:i16)
        n276 = Negate(x=w432) -> (-x=w431:i16)
        n277 = Add(x=w430, y=w431) -> (x+y=w429:i16)
        n278 = call <vilib>:"NT Write Number.vi"("Numeric"=w429, "Name"=w428) -> ()  [unwired: 9 in, 1 out]
      }
      event "Test Ring": Value Change {
        # "When a test mode helper value is selected from the ring,\nset the tree item's variable to the string value"
        n279 = event-data() -> ("NewVal"=w438:u16)  [unwired: 1 in]
        n280 = property on="Test Ring" class="Ring (strict)"() -> ("Strings []"=w439:string[])  [unwired: 2 in, 2 out]
        n281 = Index Array(array=w439, index=w438) -> (element=w437:string)
        n282 = call <vilib>:"NT Write String.vi"("String"=w437, "Name"=w436) -> ()  [unwired: 9 in, 1 out]
      }
      event "Rec Mode": Value Change {
        # "Update globals for recording mode and path to read log from.\nClear when logging and let NetworkTables set path for vision to\nuse."
        n283 = event-data() -> ("NewVal"=w450:enum32{"Stop", "Record", "Playback"})  [unwired: 1 in]
        n284 = global write "WPI_DashboardLogging Global.vi" "Logging Filename"(path "") -> ()
        n285 = global write "WPI_DashboardLogging Global.vi" "Recording"(w450) -> ()
        n286 = case shown="\"Playback\"" w450 {
          tunnel: w449 -> [_ w452 w461]
          tunnel: [_ _ w460] -> w447
          tunnel: [_ _ w459] -> _
          tunnel: w445 -> [_ _ w457]
          tunnel: cluster{i32, i32} {-250, 170} -> [_ _ w456]
          tunnel: [_ _ T24 {"Image Size"=TRUE, "Image Type"=TRUE, "Pixel Value"=TRUE, "ROI Information"=TRUE, "Zoom Factor"=FALSE} ("Image Information Shown:All Elements")] -> w440
          tunnel: [_ _ TRUE ("Zoom Factor")] -> w441
          tunnel: w443 -> [_ _ w453]
          frame Default {
          }
          frame "Stop", "Record" {
            # "Place Window too"
            n287 = invoke class="VI" method="FP.Close"(reference=w452) -> (reference out=w451:refnum<vi>)  [unwired: 2 in, 2 out]
            n288 = invoke class="VI" method="Abort VI"(reference=w451) -> ()  [unwired: 2 in, 3 out]
          }
          frame "Playback" {
            n289 = call "Open Playback Panel.vi"("Offset"=w456, "DB VI Ref"=w457, "Playback in"=w461) -> ("Playback out"=w458:refnum<vi>)  [unwired: 8 in]
            n290 = register-events(w458, w453) -> (reference out=w460:refnum<event-registration>, error out=w459:errorcluster)  [unwired: 2 in]
          }
        }
        n291 = property on="Camera Image Right" class="ImageControl"("Image Information Shown"=w440, "Image Information Visible"=w441) -> ()  [unwired: 2 in, 2 out]
        n292 = property on="Camera Image" class="ImageControl"("Image Information Shown"=w440, "Image Information Visible"=w441) -> ()  [unwired: 2 in, 2 out]
        n293 = call <vilib>:"WPI_DashboardNT Log FieldName Cache.vi"("Operation"=enum16{"Lookup/Add", "Index", "Clear"}."Clear") -> ()  [unwired: 8 in, 3 out]
      }
      event Panel Close {
        w463 = enum32{"Stop", "Record", "Playback"}."Stop" ("Rec Mode")
        # "Playback window has been closed, abort"
        n294 = event-data() -> ()  [unwired: 1 in, 4 out]
        n295 = local write "Rec Mode"(w463) -> ()
        n296 = global write "WPI_DashboardLogging Global.vi" "Recording"(w463) -> ()
      }
      event Panel Close {
        # "Abort playback window and ourself"
        n297 = event-data() -> ()  [unwired: 1 in, 4 out]
        n298 = invoke class="VI" method="FP.Close"(reference=w467) -> (reference out=w466:refnum<vi>)  [unwired: 2 in, 2 out]
        n299 = invoke class="VI" method="Abort VI"(reference=w466) -> (error out=w465:errorcluster)  [unwired: 2 in, 2 out]
        n300 = invoke class="VI" method="Abort VI"(error in=w465) -> ()  [unwired: 2 in, 3 out]
      }
      event User Event {
        n301 = event-data() -> ("IDs"=w474:cluster{"RPC field ID":u16, "Unique ID":u16}, "String"=w473:string)  [unwired: 1 in]
        n302 = Bundle("IDs"=w474, "String"=w473) -> (w472:T12)  [unwired: 1 in]
        n303 = call <vilib>:"Retrieve RPC Response.vi"("RPC Response"=w472) -> ("Output"=w470:string[][])  [unwired: 10 in]
        n304 = Build Array (concatenate)(w468, w470) -> (w469:string[][])
        n305 = local write "Command Params"(w469) -> ()
        n306 = local write "Cmd Status"("" ("Cmd Status")) -> ()
      }
      event "Tree": Double Click {
        n307 = event-data() -> ("PlatMods"=w480:T27, "Tag"=w477:string)  [unwired: 1 in]
        n308 = Unbundle(w480) -> ("Shift"=w479:bool)  [unwired: 4 out]
        n309 = String Subset(string=w477, length (rest)=1 ("length (rest)")) -> (substring=w476:string)  [unwired: 1 in]
        n310 = Not(x=w479) -> (.not. x?=w478:bool)
        n311 = case shown="\"/\"" w476 {
          tunnel: w477 -> [_ w483]
          tunnel: w478 -> [_ w482]
          frame Default {
          }
          frame "/" {
            n312 = call <vilib>:"NT Update Persistence.vi"("Persistence"=w482, "Name"=w483) -> ()  [unwired: 9 in, 1 out]
          }
        }
      }
    }
  }
  n313 = while {
    tunnel: w63 -> [w485]
    i -> [w488]
    stop <- FALSE stop-if-true
    n314 = Wait (ms)(milliseconds to wait=u32 100) -> ()  [unwired: 1 out]
    n315 = case shown="\"Playback\"" "Rec Mode" {
      tunnel: w488 -> [_ _ w503]
      tunnel: [u32 2829099 ("Base Color") u32 11141120 ("Target Color") w492] -> w484
      frame "Stop", Default {
        # "Reset the color, extra updates don't cost much"
      }
      frame "Record" {
      }
      frame "Playback" {
        # "Playback"
        n316 = Quotient & Remainder(x=w503, y=u32 50 ("milliseconds to wait")) -> (x-y*floor(x/y)=w499:u32)  [unwired: 1 out]
        n317 = Divide(x=w499, y=u32 50 ("milliseconds to wait")) -> (x/y=w496:dbl)
        n318 = Multiply(x=6.283185307179586, y=w496) -> (x*y=w501:dbl)
        n319 = Sine(x=w501) -> (sin(x)=w500:dbl)
        n320 = Absolute Value(x=w500) -> (abs(x)=w493:dbl)
        n321 = call "Interpolate RGB Color.vi"("Proportion"=w493, "Target Color"=u32 30976, "Base Color"=u32 2829099) -> ("Result Color"=w492:u32)  [unwired: 8 in]
      }
    }
    n322 = property class="Pane"(reference=w485, "PaneColor"=w484) -> ()  [unwired: 1 in, 2 out]
  }
  n323 = local write "Dashboard Tab"(T2."Drive" ("Dashboard Tab")) -> ()
  n324 = property on="On/Off" class="Bool (strict)"("Visible"=w36) -> ()  [unwired: 2 in, 2 out]
  n325 = property on="Motor" class="Clust (strict)"("Visible"=w36) -> ()  [unwired: 2 in, 2 out]
  n326 = property on="Progress" class="Clust (strict)"("Visible"=w36) -> ()  [unwired: 2 in, 2 out]
  n327 = property on="Test Ring" class="Ring (strict)"("Visible"=w36) -> ()  [unwired: 2 in, 2 out]
  n328 = property on="Rev/Fwd" class="Clust (strict)"("Visible"=w36) -> ()  [unwired: 2 in, 2 out]
  n329 = while {
    tunnel: u16 1741 ("timeout ms (25000)") -> [w505]
    stop <- FALSE stop-if-true
    n330 = TCP Create Listener(10:w505) -> (0:w504:errorcluster, 3:w506:refnum<k5>)  [unwired: 4 in, 1 out]
    n331 = case shown="No Error" w504 {
      selector: w504 -> [w508 _]
      tunnel: w506 -> [w509 _]
      frame No Error {
        n332 = while {
          tunnel: w509 -> [w512]
          tunnel: w508 -> [w511]
          stop <- FALSE stop-if-true
          n333 = TCP Wait On Listener(8:w511, 11:w512) -> (0:w513:errorcluster, 4:w514:refnum<k5>)  [unwired: 2 in, 3 out]
          n334 = local write "TCP"(w514) -> ()
          n335 = case shown="No Error" w513 {
            frame No Error {
            }
            frame Error {
              n336 = Wait (ms)(milliseconds to wait=u32 1000) -> ()  [unwired: 1 out]
            }
          }
        }
      }
      frame Error {
        n337 = Wait (ms)(milliseconds to wait=u32 1000) -> ()  [unwired: 1 out]
      }
    }
  }
  n338 = local write "Command Selection"(u16 0 ("milliseconds to wait")) -> ()
  n339 = local write "Command Params"(string[][] [] ("Command Params")) -> ()
  n340 = global write "WPI_DashboardLogging Global.vi" "Recording"(w57) -> ()
  n341 = local write "Rec Mode"(w57) -> ()
  n342 = call <vilib>:"NT Write String.vi"("String"="Select Auto", "Name"="Auto Selector") -> ()  [unwired: 9 in, 1 out]
  n343 = while {
    stop <- FALSE stop-if-true
    w520 = path "C:/3654Programming" ("base path")
    n344 = First Call?() -> (First Call?: T/F=w551:bool)
    n345 = case shown="\"Competition\", Default" "ConfigFile" {
      tunnel: ["Competition.ini" "Sister.ini" "DrivePractice.ini"] -> w547
      frame "Competition", Default {
      }
      frame "Sister" {
      }
      frame "DrivePractice" {
      }
    }
    n346 = Select(t=TRUE, s=w551, f="Load") -> (s? t:f=w558:bool)
    n347 = call-poly <vilib>:"NT Write Value.vi"("Numeric"="ConfigFile", "Name"="ConfigFile") -> ()  [unwired: 9 in, 1 out]
    n348 = Select(t=1.0, s=w558, f=0.0) -> (s? t:f=w557:dbl)
    n349 = Select(t=2.0, s="Save", f=w557) -> (s? t:f=w549:dbl)
    n350 = call-poly <vilib>:"NT Write Value.vi"("Numeric"="DriveMode", "Name"="DriveMode") -> ()  [unwired: 9 in, 1 out]
    n351 = Build Path(base path=w520, name or relative path=w547) -> (appended path=w546:path)
    n352 = case shown="1" w549 {
      tunnel: w546 -> [_ w693 w697]
      tunnel: "FTeleLeft" -> [_ w650 w722]
      tunnel: "FTeleRight" -> [_ w649 w721]
      tunnel: "PTele" -> [_ w648 w720]
      tunnel: "ITele" -> [_ w647 w719]
      tunnel: "DTele" -> [_ w646 w718]
      tunnel: "FAutoLeft" -> [_ w645 w717]
      tunnel: "FAutoRight" -> [_ w644 w716]
      tunnel: "PAuto" -> [_ w643 w715]
      tunnel: "IAuto" -> [_ w642 w714]
      tunnel: "DAuto" -> [_ w641 w713]
      tunnel: "FTeleGyro" -> [_ w607 w712]
      tunnel: "PTeleGyro" -> [_ w606 w711]
      tunnel: "ITeleGyro" -> [_ w605 w710]
      tunnel: "DTeleGyro" -> [_ w604 w709]
      tunnel: "FAutoGyro" -> [_ w603 w708]
      tunnel: "PAutoGyro" -> [_ w602 w707]
      tunnel: "IAutoGyro" -> [_ w601 w706]
      tunnel: "DAutoGyro" -> [_ w600 w705]
      tunnel: "RampRateAuto" -> [_ w596 w704]
      tunnel: "RampRateTele" -> [_ w595 w703]
      tunnel: "XYRatio" -> [_ w594 w702]
      tunnel: "DriveMaxRPM" -> [_ w572 w700]
      tunnel: "TurboPercent" -> [_ w571 w699]
      tunnel: "NormalPercent" -> [_ w570 w698]
      tunnel: "DriveMode" -> [_ w564 w695]
      tunnel: w520 -> [_ _ w696]
      frame 0, Default {
        # "default dashboard code should be running variables in basic/custom tabs to network tables.\nshould probably leave this area blank."
      }
      frame 1 {
        w569 = "Drive"
        w617 = "Gyro" ("section")
        w661 = "AutoPIDF" ("section")
        w677 = "TelePIDF" ("section")
        # "To create the local variables do this:  Right-click variable name > create > local variable"
        # "load: loads ini file(s)\nwe will have a different ini file for each robot."
        n353 = call <vilib>:"Open Config Data.vi"("create file if necessary (T)"=TRUE, "configuration file path"=w693) -> ("error out"=w691:errorcluster, "refnum"=w692:T28)  [unwired: 7 in, 1 out]
        n354 = call-poly <vilib>:"Read Key.vi"("section"=w677, "error in (no error)"=w691, "default value"=w650, "key"="FTeleLeft", "refnum"=w692) -> ("error out"=w688:errorcluster, "value"=w676:dbl, "refnum out"=w689:T28)  [unwired: 3 in, 1 out]
        n355 = local write "FTeleLeft"(w676) -> ()
        n356 = call-poly <vilib>:"Read Key.vi"("section"=w677, "error in (no error)"=w688, "default value"=w649, "key"="FTeleRight", "refnum"=w689) -> ("error out"=w686:errorcluster, "value"=w675:dbl, "refnum out"=w687:T28)  [unwired: 3 in, 1 out]
        n357 = local write "FTeleRight"(w675) -> ()
        n358 = call-poly <vilib>:"Read Key.vi"("section"=w677, "error in (no error)"=w686, "default value"=w648, "key"="PTele", "refnum"=w687) -> ("error out"=w684:errorcluster, "value"=w674:dbl, "refnum out"=w685:T28)  [unwired: 3 in, 1 out]
        n359 = local write "PTele"(w674) -> ()
        n360 = call-poly <vilib>:"Read Key.vi"("section"=w677, "error in (no error)"=w684, "default value"=w647, "key"="ITele", "refnum"=w685) -> ("error out"=w682:errorcluster, "value"=w673:dbl, "refnum out"=w683:T28)  [unwired: 3 in, 1 out]
        n361 = local write "ITele"(w673) -> ()
        n362 = call-poly <vilib>:"Read Key.vi"("section"=w677, "error in (no error)"=w682, "default value"=w646, "key"="DTele", "refnum"=w683) -> ("error out"=w666:errorcluster, "value"=w672:dbl, "refnum out"=w671:T28)  [unwired: 3 in, 1 out]
        n363 = call-poly <vilib>:"Read Key.vi"("section"=w661, "error in (no error)"=w666, "default value"=w645, "key"="FAutoLeft", "refnum"=w671) -> ("error out"=w665:errorcluster, "value"=w655:dbl, "refnum out"=w670:T28)  [unwired: 3 in, 1 out]
        n364 = local write "FAutoLeft"(w655) -> ()
        n365 = call-poly <vilib>:"Read Key.vi"("section"=w661, "error in (no error)"=w665, "default value"=w644, "key"="FAutoRight", "refnum"=w670) -> ("error out"=w664:errorcluster, "value"=w654:dbl, "refnum out"=w669:T28)  [unwired: 3 in, 1 out]
        n366 = local write "FAutoRight"(w654) -> ()
        n367 = call-poly <vilib>:"Read Key.vi"("section"=w661, "error in (no error)"=w664, "default value"=w643, "key"="PAuto", "refnum"=w669) -> ("error out"=w663:errorcluster, "value"=w653:dbl, "refnum out"=w668:T28)  [unwired: 3 in, 1 out]
        n368 = local write "PAuto"(w653) -> ()
        n369 = call-poly <vilib>:"Read Key.vi"("section"=w661, "error in (no error)"=w663, "default value"=w642, "key"="IAuto", "refnum"=w668) -> ("error out"=w662:errorcluster, "value"=w652:dbl, "refnum out"=w667:T28)  [unwired: 3 in, 1 out]
        n370 = local write "IAuto"(w652) -> ()
        n371 = call-poly <vilib>:"Read Key.vi"("section"=w661, "error in (no error)"=w662, "default value"=w641, "key"="DAuto", "refnum"=w667) -> ("error out"=w639:errorcluster, "value"=w651:dbl, "refnum out"=w640:T28)  [unwired: 3 in, 1 out]
        n372 = call-poly <vilib>:"Read Key.vi"("section"=w617, "error in (no error)"=w639, "default value"=w607, "key"="FTeleGyro", "refnum"=w640) -> ("error out"=w636:errorcluster, "value"=w615:dbl, "refnum out"=w637:T28)  [unwired: 3 in, 1 out]
        n373 = local write "FTeleGyro"(w615) -> ()
        n374 = call-poly <vilib>:"Read Key.vi"("section"=w617, "error in (no error)"=w636, "default value"=w606, "key"="PTeleGyro", "refnum"=w637) -> ("error out"=w633:errorcluster, "value"=w614:dbl, "refnum out"=w634:T28)  [unwired: 3 in, 1 out]
        n375 = local write "PTeleGyro"(w614) -> ()
        n376 = call-poly <vilib>:"Read Key.vi"("section"=w617, "error in (no error)"=w633, "default value"=w605, "key"="ITeleGyro", "refnum"=w634) -> ("error out"=w630:errorcluster, "value"=w613:dbl, "refnum out"=w631:T28)  [unwired: 3 in, 1 out]
        n377 = local write "ITeleGyro"(w613) -> ()
        n378 = call-poly <vilib>:"Read Key.vi"("section"=w617, "error in (no error)"=w630, "default value"=w604, "key"="DTeleGyro", "refnum"=w631) -> ("error out"=w627:errorcluster, "value"=w612:dbl, "refnum out"=w628:T28)  [unwired: 3 in, 1 out]
        n379 = local write "DTeleGyro"(w612) -> ()
        n380 = local write "DAuto"(w651) -> ()
        n381 = call-poly <vilib>:"Read Key.vi"("section"=w617, "error in (no error)"=w627, "default value"=w603, "key"="FAutoGyro", "refnum"=w628) -> ("error out"=w624:errorcluster, "value"=w611:dbl, "refnum out"=w625:T28)  [unwired: 3 in, 1 out]
        n382 = local write "FAutoGyro"(w611) -> ()
        n383 = local write "DTele"(w672) -> ()
        n384 = call-poly <vilib>:"Read Key.vi"("section"=w617, "error in (no error)"=w624, "default value"=w602, "key"="PAutoGyro", "refnum"=w625) -> ("error out"=w621:errorcluster, "value"=w610:dbl, "refnum out"=w622:T28)  [unwired: 3 in, 1 out]
        n385 = local write "PAutoGyro"(w610) -> ()
        n386 = call-poly <vilib>:"Read Key.vi"("section"=w617, "error in (no error)"=w621, "default value"=w601, "key"="IAutoGyro", "refnum"=w622) -> ("error out"=w618:errorcluster, "value"=w609:dbl, "refnum out"=w619:T28)  [unwired: 3 in, 1 out]
        n387 = local write "IAutoGyro"(w609) -> ()
        n388 = call-poly <vilib>:"Read Key.vi"("section"=w617, "error in (no error)"=w618, "default value"=w600, "key"="DAutoGyro", "refnum"=w619) -> ("error out"=w585:errorcluster, "value"=w608:dbl, "refnum out"=w591:T28)  [unwired: 3 in, 1 out]
        n389 = call-poly <vilib>:"Read Key.vi"("section"=w569, "error in (no error)"=w585, "default value"=w596, "key"="RampRateAuto", "refnum"=w591) -> ("error out"=w593:errorcluster, "value"=w588:dbl, "refnum out"=w590:T28)  [unwired: 3 in, 1 out]
        n390 = local write "RampRateAuto"(w588) -> ()
        n391 = call-poly <vilib>:"Read Key.vi"("section"=w569, "error in (no error)"=w593, "default value"=w595, "key"="RampRateTele", "refnum"=w590) -> ("error out"=w592:errorcluster, "value"=w587:dbl, "refnum out"=w589:T28)  [unwired: 3 in, 1 out]
        n392 = local write "RampRateTele"(w587) -> ()
        n393 = call-poly <vilib>:"Read Key.vi"("section"=w569, "error in (no error)"=w592, "default value"=w594, "key"="XYRatio", "refnum"=w589) -> ("error out"=w581:errorcluster, "value"=w586:dbl, "refnum out"=w578:T28)  [unwired: 3 in, 1 out]
        n394 = local write "XYRatio"(w586) -> ()
        n395 = call-poly <vilib>:"Read Key.vi"("section"=w569, "error in (no error)"=w581, "default value"=w572, "key"="DriveMaxRPM", "refnum"=w578) -> ("error out"=w580:errorcluster, "value"=w575:dbl, "refnum out"=w577:T28)  [unwired: 3 in, 1 out]
        n396 = local write "DriveMaxRPM"(w575) -> ()
        n397 = call-poly <vilib>:"Read Key.vi"("section"=w569, "error in (no error)"=w580, "default value"=w571, "key"="TurboPercent", "refnum"=w577) -> ("error out"=w579:errorcluster, "value"=w574:dbl, "refnum out"=w576:T28)  [unwired: 3 in, 1 out]
        n398 = local write "TurboPercent"(w574) -> ()
        n399 = call-poly <vilib>:"Read Key.vi"("section"=w569, "error in (no error)"=w579, "default value"=w570, "key"="NormalPercent", "refnum"=w576) -> ("error out"=w567:errorcluster, "value"=w573:dbl, "refnum out"=w566:T28)  [unwired: 3 in, 1 out]
        n400 = local write "NormalPercent"(w573) -> ()
        n401 = local write "DAutoGyro"(w608) -> ()
        n402 = call-poly <vilib>:"Read Key.vi"("section"=w569, "error in (no error)"=w567, "default value"=w564, "key"="DriveMode", "refnum"=w566) -> ("error out"=w563:errorcluster, "value"=w565:i32, "refnum out"=w562:T28)  [unwired: 3 in, 1 out]
        n403 = local write "DriveMode"(w565) -> ()
        n404 = call <vilib>:"Close Config Data.vi"("error in (no error)"=w563, "refnum"=w562) -> ()  [unwired: 8 in, 2 out]
      }
      frame 2 {
        w737 = "Drive"
        w756 = "Gyro" ("section")
        w785 = "AutoPIDF" ("section")
        w796 = "TelePIDF" ("section")
        # "To create the local variables do this:  Right-click variable name > create > local variable"
        # "load: loads ini file(s)\nwe will have a different ini file for each robot."
        n405 = call <vilib>:"Open Config Data.vi"("create file if necessary (T)"=TRUE, "configuration file path"=w697) -> ("error out"=w810:errorcluster, "refnum"=w811:T28)  [unwired: 7 in, 1 out]
        n406 = call-poly <vilib>:"Write Key.vi"("section"=w796, "error in (no error)"=w810, "value"=w722, "key"="FTeleLeft", "refnum"=w811) -> ("error out"=w807:errorcluster, "refnum out"=w808:T28)  [unwired: 4 in, 1 out]
        n407 = call-poly <vilib>:"Write Key.vi"("section"=w796, "error in (no error)"=w807, "value"=w721, "key"="FTeleRight", "refnum"=w808) -> ("error out"=w805:errorcluster, "refnum out"=w806:T28)  [unwired: 4 in, 1 out]
        n408 = call-poly <vilib>:"Write Key.vi"("section"=w796, "error in (no error)"=w805, "value"=w720, "key"="PTele", "refnum"=w806) -> ("error out"=w803:errorcluster, "refnum out"=w804:T28)  [unwired: 4 in, 1 out]
        n409 = call-poly <vilib>:"Write Key.vi"("section"=w796, "error in (no error)"=w803, "value"=w719, "key"="ITele", "refnum"=w804) -> ("error out"=w801:errorcluster, "refnum out"=w802:T28)  [unwired: 4 in, 1 out]
        n410 = call-poly <vilib>:"Write Key.vi"("section"=w796, "error in (no error)"=w801, "value"=w718, "key"="DTele", "refnum"=w802) -> ("error out"=w790:errorcluster, "refnum out"=w795:T28)  [unwired: 4 in, 1 out]
        n411 = call-poly <vilib>:"Write Key.vi"("section"=w785, "error in (no error)"=w790, "value"=w717, "key"="FAutoLeft", "refnum"=w795) -> ("error out"=w789:errorcluster, "refnum out"=w794:T28)  [unwired: 4 in, 1 out]
        n412 = call-poly <vilib>:"Write Key.vi"("section"=w785, "error in (no error)"=w789, "value"=w716, "key"="FAutoRight", "refnum"=w794) -> ("error out"=w788:errorcluster, "refnum out"=w793:T28)  [unwired: 4 in, 1 out]
        n413 = call-poly <vilib>:"Write Key.vi"("section"=w785, "error in (no error)"=w788, "value"=w715, "key"="PAuto", "refnum"=w793) -> ("error out"=w787:errorcluster, "refnum out"=w792:T28)  [unwired: 4 in, 1 out]
        n414 = call-poly <vilib>:"Write Key.vi"("section"=w785, "error in (no error)"=w787, "value"=w714, "key"="IAuto", "refnum"=w792) -> ("error out"=w786:errorcluster, "refnum out"=w791:T28)  [unwired: 4 in, 1 out]
        n415 = call-poly <vilib>:"Write Key.vi"("section"=w785, "error in (no error)"=w786, "value"=w713, "key"="DAuto", "refnum"=w791) -> ("error out"=w778:errorcluster, "refnum out"=w779:T28)  [unwired: 4 in, 1 out]
        n416 = call-poly <vilib>:"Write Key.vi"("section"=w756, "error in (no error)"=w778, "value"=w712, "key"="FTeleGyro", "refnum"=w779) -> ("error out"=w775:errorcluster, "refnum out"=w776:T28)  [unwired: 4 in, 1 out]
        n417 = call-poly <vilib>:"Write Key.vi"("section"=w756, "error in (no error)"=w775, "value"=w711, "key"="PTeleGyro", "refnum"=w776) -> ("error out"=w772:errorcluster, "refnum out"=w773:T28)  [unwired: 4 in, 1 out]
        n418 = call-poly <vilib>:"Write Key.vi"("section"=w756, "error in (no error)"=w772, "value"=w710, "key"="ITeleGyro", "refnum"=w773) -> ("error out"=w769:errorcluster, "refnum out"=w770:T28)  [unwired: 4 in, 1 out]
        n419 = call-poly <vilib>:"Write Key.vi"("section"=w756, "error in (no error)"=w769, "value"=w709, "key"="DTeleGyro", "refnum"=w770) -> ("error out"=w766:errorcluster, "refnum out"=w767:T28)  [unwired: 4 in, 1 out]
        n420 = call-poly <vilib>:"Write Key.vi"("section"=w756, "error in (no error)"=w766, "value"=w708, "key"="FAutoGyro", "refnum"=w767) -> ("error out"=w763:errorcluster, "refnum out"=w764:T28)  [unwired: 4 in, 1 out]
        n421 = call-poly <vilib>:"Write Key.vi"("section"=w756, "error in (no error)"=w763, "value"=w707, "key"="PAutoGyro", "refnum"=w764) -> ("error out"=w760:errorcluster, "refnum out"=w761:T28)  [unwired: 4 in, 1 out]
        n422 = Get Date/Time In Seconds() -> (seconds since 1Jan1904=w731:timestamp)
        n423 = call-poly <vilib>:"Write Key.vi"("section"=w756, "error in (no error)"=w760, "value"=w706, "key"="IAutoGyro", "refnum"=w761) -> ("error out"=w757:errorcluster, "refnum out"=w758:T28)  [unwired: 4 in, 1 out]
        n424 = Format Date/Time String(time format string (%c)="%y%m%d_%H%M%S", seconds (now)=w731) -> (date/time string=w728:string)  [unwired: 1 in]
        n425 = call-poly <vilib>:"Write Key.vi"("section"=w756, "error in (no error)"=w757, "value"=w705, "key"="DAutoGyro", "refnum"=w758) -> ("error out"=w746:errorcluster, "refnum out"=w749:T28)  [unwired: 4 in, 1 out]
        n426 = call-poly <vilib>:"Write Key.vi"("section"=w737, "error in (no error)"=w746, "value"=w704, "key"="RampRateAuto", "refnum"=w749) -> ("error out"=w751:errorcluster, "refnum out"=w748:T28)  [unwired: 4 in, 1 out]
        n427 = call-poly <vilib>:"Write Key.vi"("section"=w737, "error in (no error)"=w751, "value"=w703, "key"="RampRateTele", "refnum"=w748) -> ("error out"=w750:errorcluster, "refnum out"=w747:T28)  [unwired: 4 in, 1 out]
        n428 = call-poly <vilib>:"Write Key.vi"("section"=w737, "error in (no error)"=w750, "value"=w702, "key"="XYRatio", "refnum"=w747) -> ("error out"=w701:errorcluster, "refnum out"=w740:T28)  [unwired: 4 in, 1 out]
        n429 = call-poly <vilib>:"Write Key.vi"("section"=w737, "error in (no error)"=w701, "value"=w700, "key"="DriveMaxRPM", "refnum"=w740) -> ("error out"=w742:errorcluster, "refnum out"=w739:T28)  [unwired: 4 in, 1 out]
        n430 = call-poly <vilib>:"Write Key.vi"("section"=w737, "error in (no error)"=w742, "value"=w699, "key"="TurboPercent", "refnum"=w739) -> ("error out"=w741:errorcluster, "refnum out"=w738:T28)  [unwired: 4 in, 1 out]
        n431 = call-poly <vilib>:"Write Key.vi"("section"=w737, "error in (no error)"=w741, "value"=w698, "key"="NormalPercent", "refnum"=w738) -> ("error out"=w735:errorcluster, "refnum out"=w734:T28)  [unwired: 4 in, 1 out]
        n432 = Concatenate Strings("WrightDashArchive" ("string"), "_" ("string"), w728) -> (w726:string)
        n433 = call-poly <vilib>:"Write Key.vi"("section"=w737, "error in (no error)"=w735, "value"=w695, "key"="DriveMode", "refnum"=w734) -> ("error out"=w733:errorcluster, "refnum out"=w732:T28)  [unwired: 4 in, 1 out]
        n434 = Build Path(base path=w696, name or relative path=w726) -> (appended path=w725:path)
        n435 = call <vilib>:"Close Config Data.vi"("error in (no error)"=w733, "refnum"=w732) -> ("error out"=w724:errorcluster)  [unwired: 8 in, 1 out]
        n436 = Create Folder(path (use dialog)=w725, error in=w724) -> (error out=w723:errorcluster)  [unwired: 1 in, 2 out]
        n437 = Copy(8:w723, 10:w725, 11:w697) -> ()  [unwired: 2 in, 3 out]
      }
    }
  }
  n438 = while {
    stop <- FALSE stop-if-true
    n439 = case shown="True" TRUE {
      frame False {
      }
      frame True {
        # "All drive tab. none saved to ini."
        n440 = call-poly <vilib>:"NT Write Value.vi"("Boolean"="Boolean 2", "Name"="Boolean 2") -> ()  [unwired: 9 in, 1 out]
        n441 = call-poly <vilib>:"NT Write Value.vi"("Numeric"="RobotPosition", "Name"="RobotPosition") -> ()  [unwired: 9 in, 1 out]
        n442 = call-poly <vilib>:"NT Write Value.vi"("Numeric"="Encoders", "Name"="Encoders") -> ()  [unwired: 9 in, 1 out]
        n443 = call-poly <vilib>:"NT Write Value.vi"("Boolean"="Logging", "Name"="Logging") -> ()  [unwired: 9 in, 1 out]
        n444 = call-poly <vilib>:"NT Write Value.vi"("Numeric"="Autonomous", "Name"="Autonomous") -> ()  [unwired: 9 in, 1 out]
        n445 = call-poly <vilib>:"NT Write Value.vi"("Boolean"="Gyro", "Name"="Gyro") -> ()  [unwired: 9 in, 1 out]
      }
    }
    n446 = Wait (ms)(milliseconds to wait=u32 50) -> ()  [unwired: 1 out]
  }
